vi "ConfigurationFileWriteCase.vi"() -> ()   [LabVIEW 2016]
uses:
  <vilib>/Utility/config.llb/NI_LVConfig.lvlib
  <vilib>/Utility/config.llb/Write Key (String).vi
  <vilib>/Utility/config.llb/Write Key (Boolean).vi
  <vilib>/Utility/config.llb/Write Key (Path).vi
  <vilib>/Utility/config.llb/Write Key (Double).vi
  controls/Enum.ctl
  <vilib>/Utility/config.llb/Write Key (U32).vi
  <vilib>/Utility/config.llb/Write Key (I32).vi
panel:
  in  "default name":path=path "Configuration File3.ini"
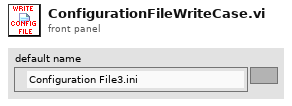
[diagram p1: front panel]
types:
  T1 = enum16{"General", "WindowPositions", "Calibration", "ZController", "Motor", "Waveforns", "ScanControl", "ScanMonitor", "Signals", "Ramp"}
  T2 = typedef "NI_LVConfig.lvlib/Config Data RefNum.ctl" = refnum<k1>
  T3 = typedef "Enum.ctl" = enum16{"Init", "Read", "Write"}
  T4 = enum16{"fractional", "engineering", "exponential"}
  T5 = enum16{"Vert. Deflection", "Horiz. Deflection", "Amplitude", "..."}
  T6 = enum32{"No Selection", "FullScale", "Standard Deviation"}
  T7 = cluster{i32, "Direction":enum16{"Forward", "Backward"}, "Processing":enum16{"None", "Offset", "Line", "Polynom"}, "Color":enum16{"Blue", "Gray", "Gold", "Green", "Red", "Asylum", "Adrian", "Nanoscope", "NanoscopeIII"}}
  T8 = enum32{"Invalid", "Standard", "Closed", "Hidden", "Minimized", "Maximized"}
  T9 = typedef "LVPositionTypeDef.ctl" = cluster{"Left":i32, "Top":i32}
  T10 = cluster{"calibName":string[], "calibParameters":cluster{"Sensitivity":cluster{"Sens X":dbl, "Sens Y":dbl, "Sens Z":dbl}, "Range":cluster{"Range X":dbl, "Range Y":dbl, "Range Z":dbl}, "HV gain":cluster{"HV gain X":dbl, "HV gain Y":dbl, "HV gain Z":dbl}}[], "calibIndex":i32}
  T11 = cluster{"Sensitivity":cluster{"Sens X":dbl, "Sens Y":dbl, "Sens Z":dbl}, "Range":cluster{"Range X":dbl, "Range Y":dbl, "Range Z":dbl}, "HV gain":cluster{"HV gain X":dbl, "HV gain Y":dbl, "HV gain Z":dbl}}[]
  T12 = cluster{"Sensitivity":cluster{"Sens X":dbl, "Sens Y":dbl, "Sens Z":dbl}, "Range":cluster{"Range X":dbl, "Range Y":dbl, "Range Z":dbl}, "HV gain":cluster{"HV gain X":dbl, "HV gain Y":dbl, "HV gain Z":dbl}}
  T13 = cluster{"Sens X":dbl, "Sens Y":dbl, "Sens Z":dbl}
  T14 = cluster{"Range X":dbl, "Range Y":dbl, "Range Z":dbl}
  T15 = cluster{"HV gain X":dbl, "HV gain Y":dbl, "HV gain Z":dbl}
  T16 = cluster{"ActiveController":dbl, "ControllerNames":string[], "ControllerParameters":cluster{"Controller Config":cluster{"Slope":bool, "Controller type":enum16{"Bipolar", "Absolute"}, "Controller name":string, "Control Signal name":string, "Signal":enum16{"Vert. Deflection", "Horiz. Deflection", "Amplitude", "..."}, "Unit":string}, "PID":cluster{"Setpoint":dbl, "P Gain":dbl, "I Gain":dbl}}[]}
  T17 = cluster{"Controller Config":cluster{"Slope":bool, "Controller type":enum16{"Bipolar", "Absolute"}, "Controller name":string, "Control Signal name":string, "Signal":enum16{"Vert. Deflection", "Horiz. Deflection", "Amplitude", "..."}, "Unit":string}, "PID":cluster{"Setpoint":dbl, "P Gain":dbl, "I Gain":dbl}}[]
  T18 = cluster{"Slope":bool, "Controller type":enum16{"Bipolar", "Absolute"}, "Controller name":string, "Control Signal name":string, "Signal":enum16{"Vert. Deflection", "Horiz. Deflection", "Amplitude", "..."}, "Unit":string}
  T19 = cluster{"Setpoint":dbl, "P Gain":dbl, "I Gain":dbl}
  T20 = typedef "ScanWaveform.ctl" = enum16{"Sine Wave", "Triangle Wave", "Rounded Wave"}
  T21 = cluster{"slowWavePts":u16, "fastWavePts":u16, "slowWaveType":T20, "fastWaveType":T20, "slowRoundPts":u16, "fastRoundPts":u16, "singleDirectionScan":bool}
  T22 = cluster{"Width":dbl, "Height":dbl, "X Offset":dbl, "Y Offset":dbl, "Angle":dbl, "Pixels/Line":u16, "Lines":u16, "Time/Line":dbl, "Scan Rate":dbl}
  T23 = enum16{"Blue", "Gray", "Gold", "Green", "Red", "Asylum", "Adrian", "Nanoscope", "NanoscopeIII"}
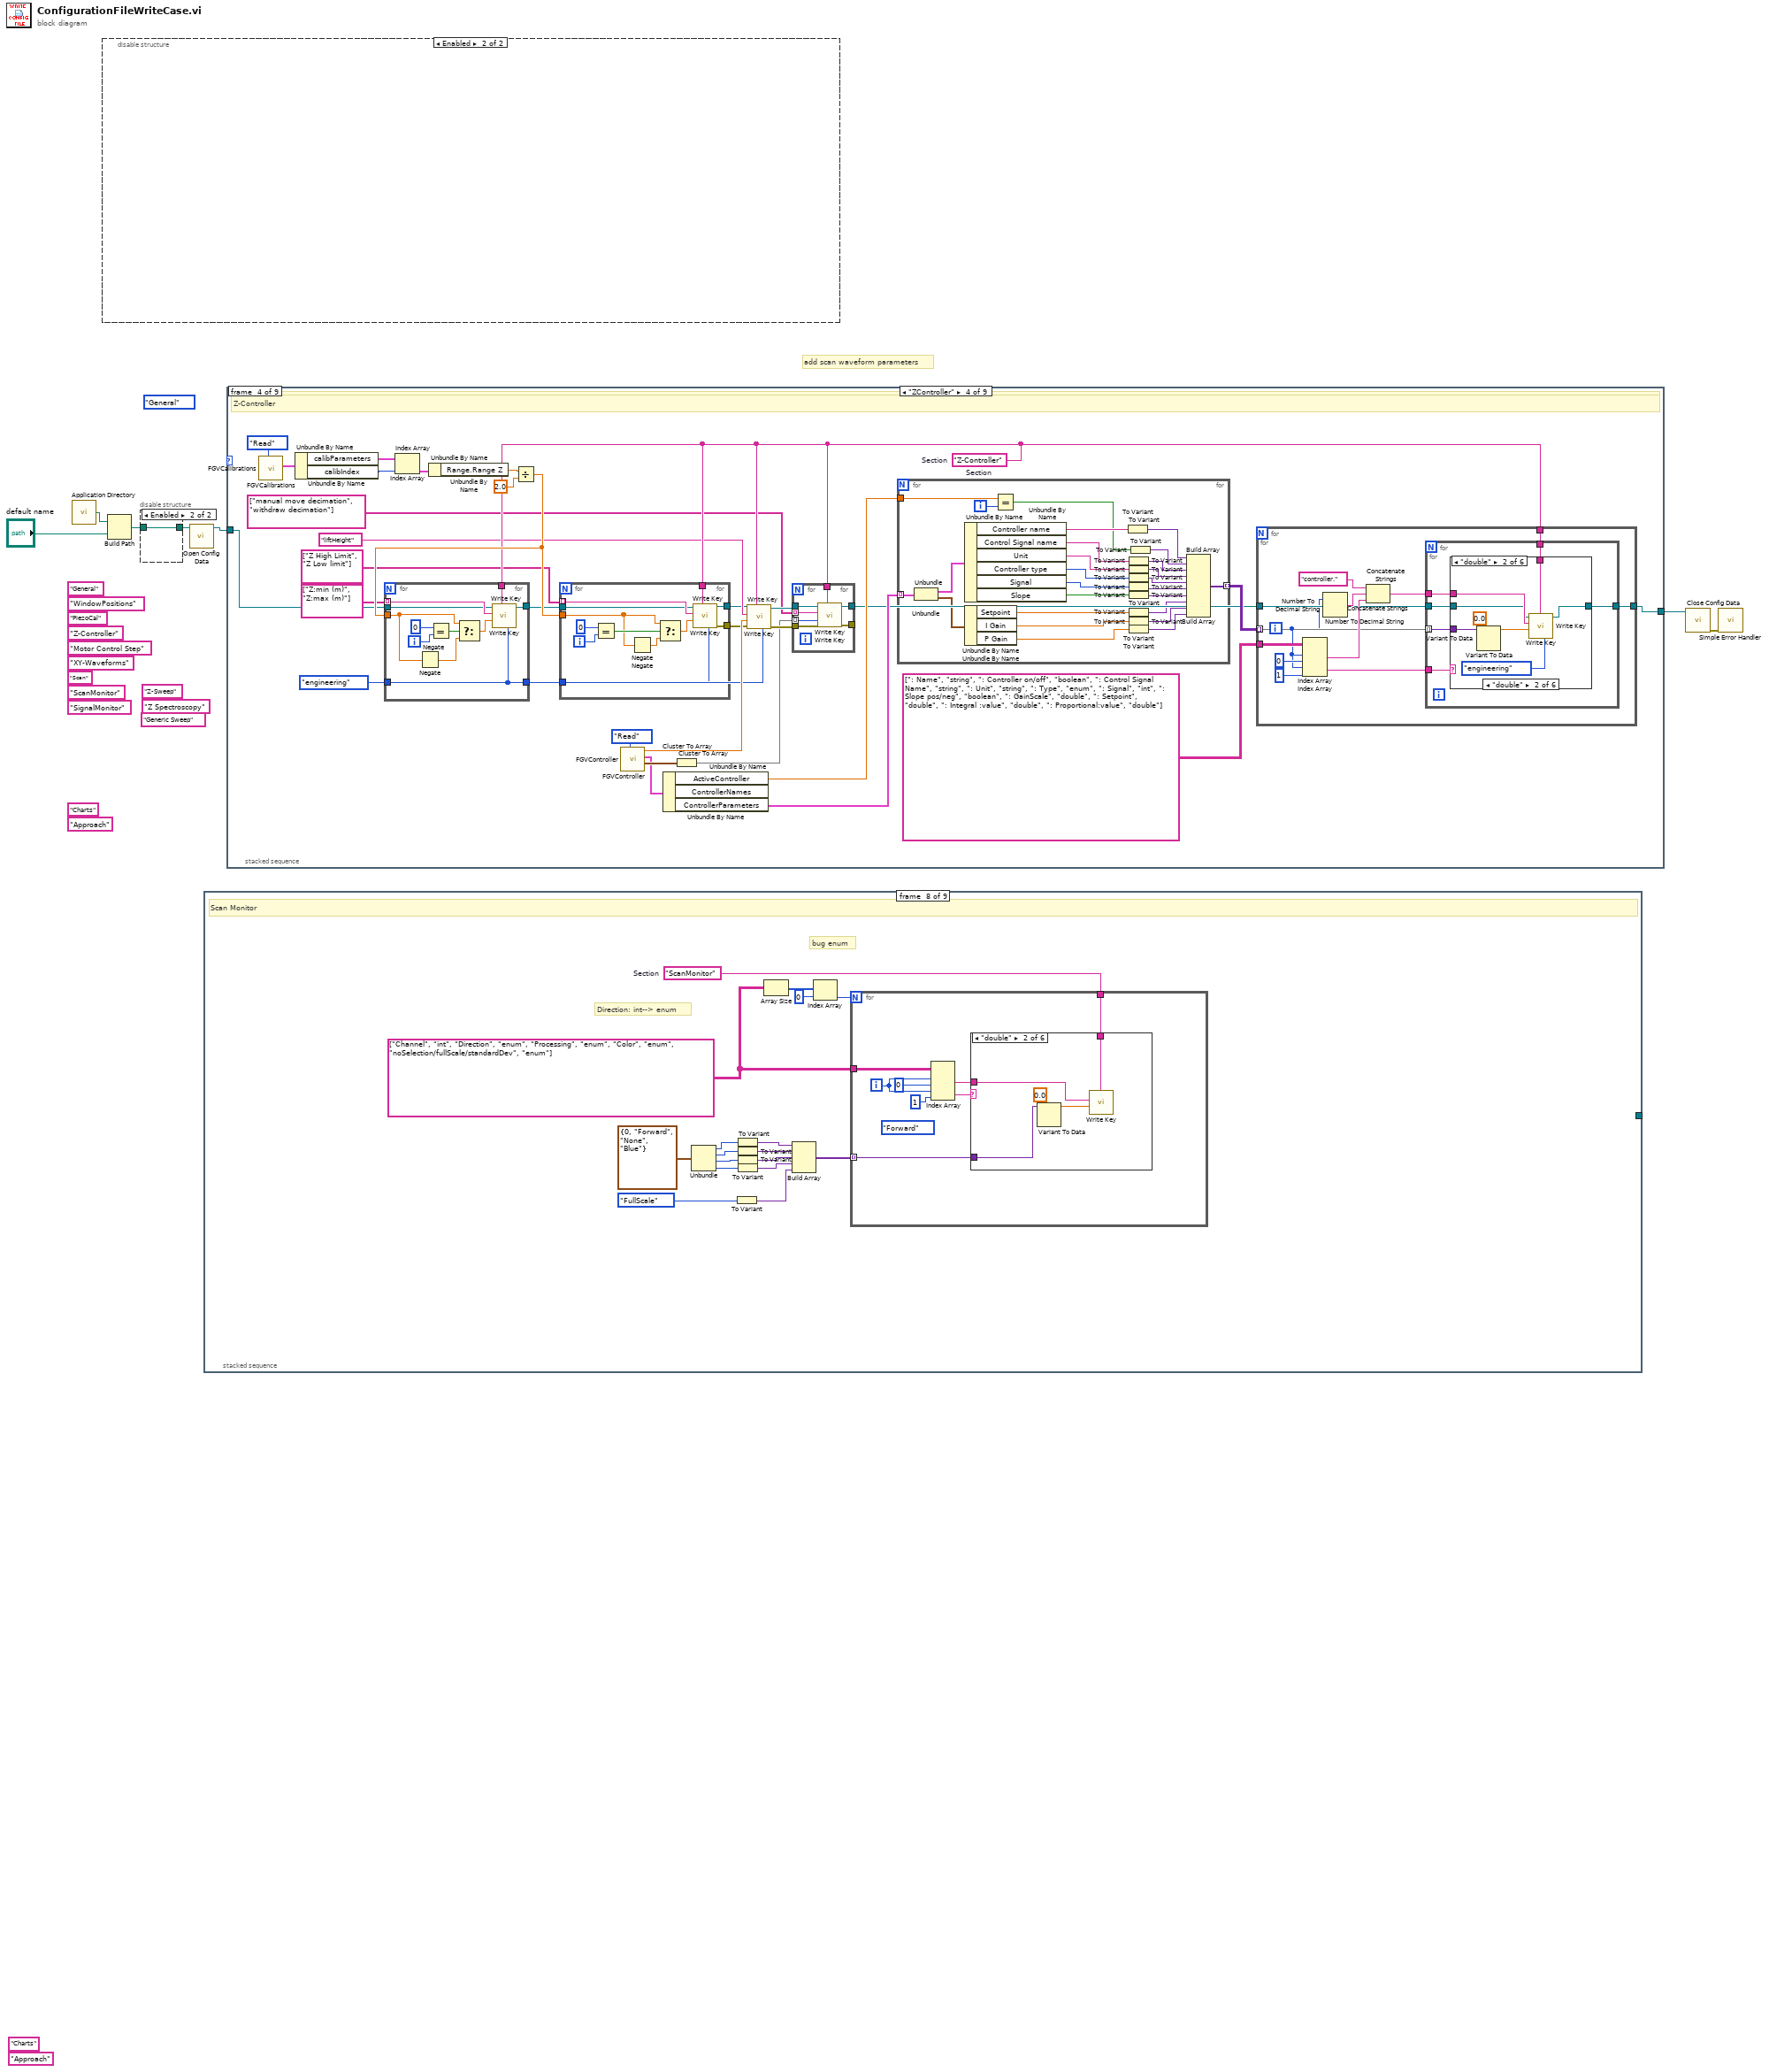
[diagram p0: block diagram]
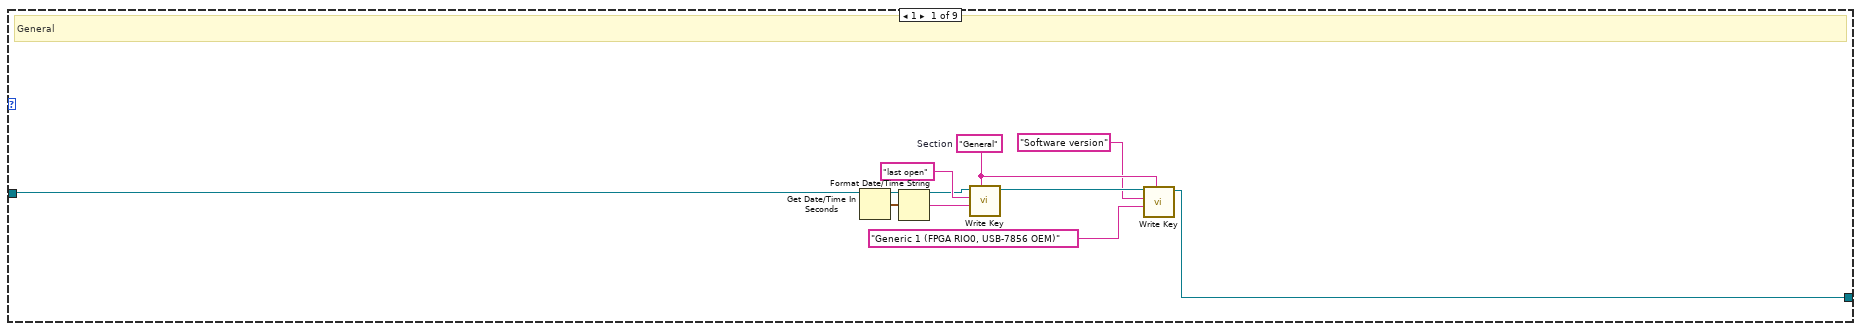
[diagram p2: hidden frame]
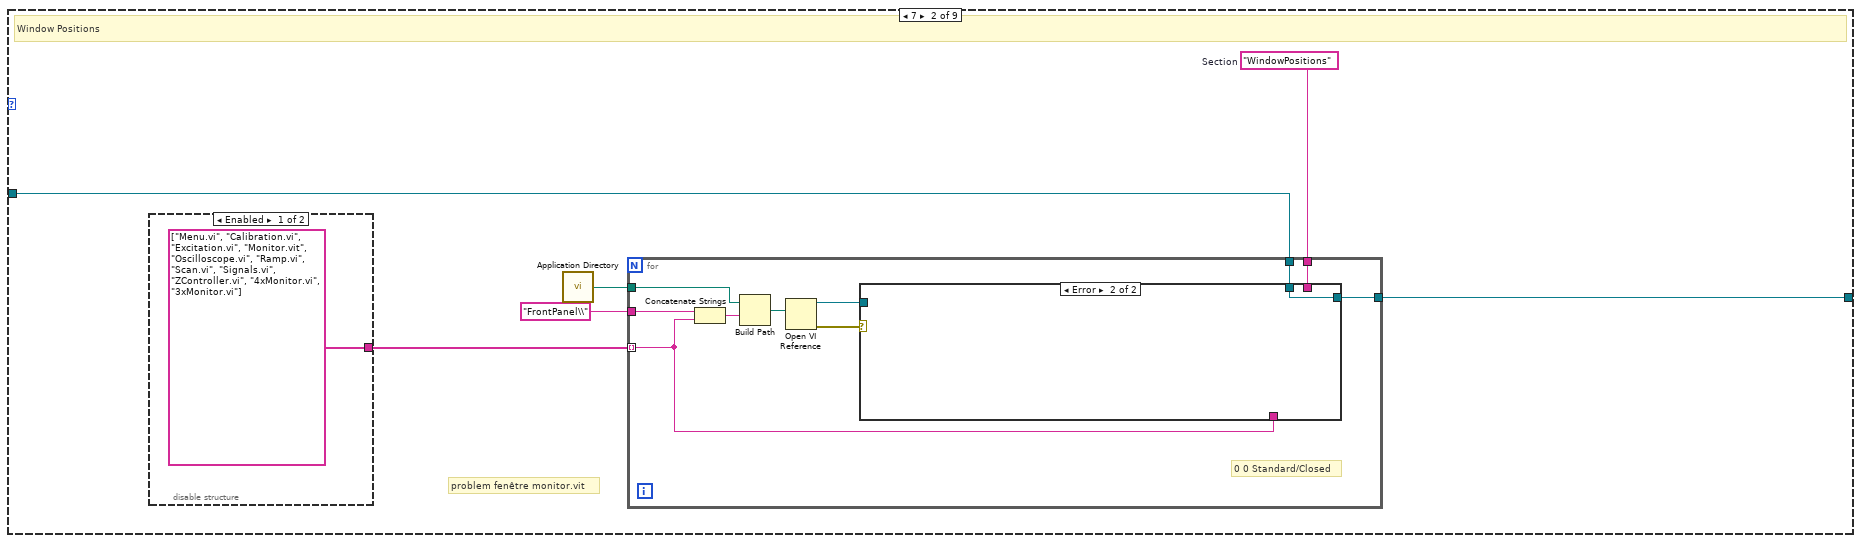
[diagram p3: hidden frame]
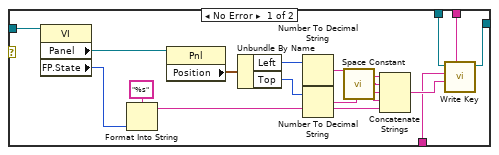
[diagram p5: hidden frame]
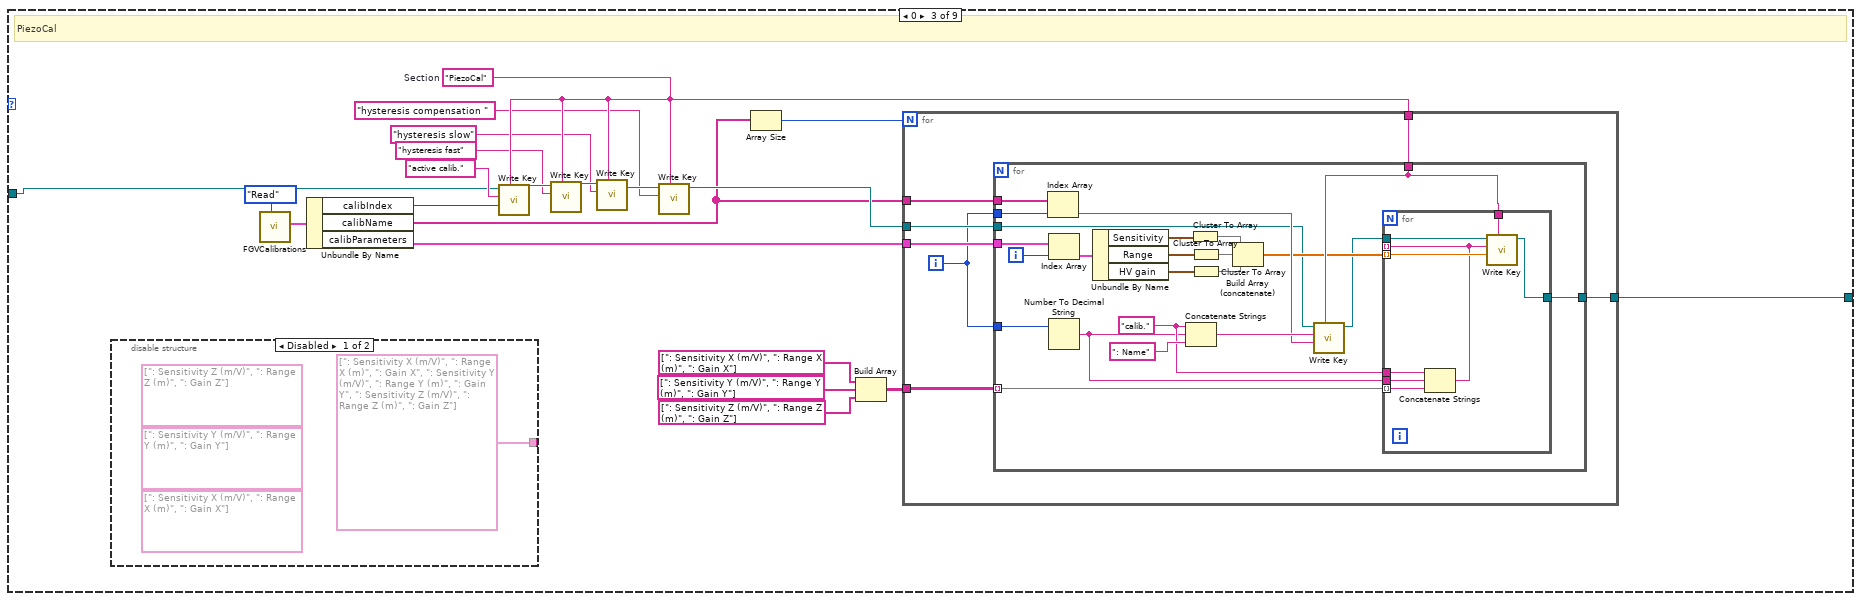
[diagram p6: hidden frame]
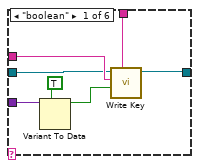
[diagram p8: hidden frame]
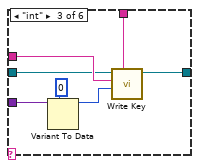
[diagram p9: hidden frame]
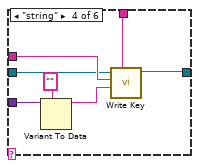
[diagram p10: hidden frame]
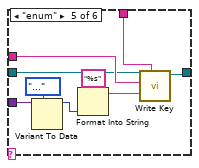
[diagram p11: hidden frame]
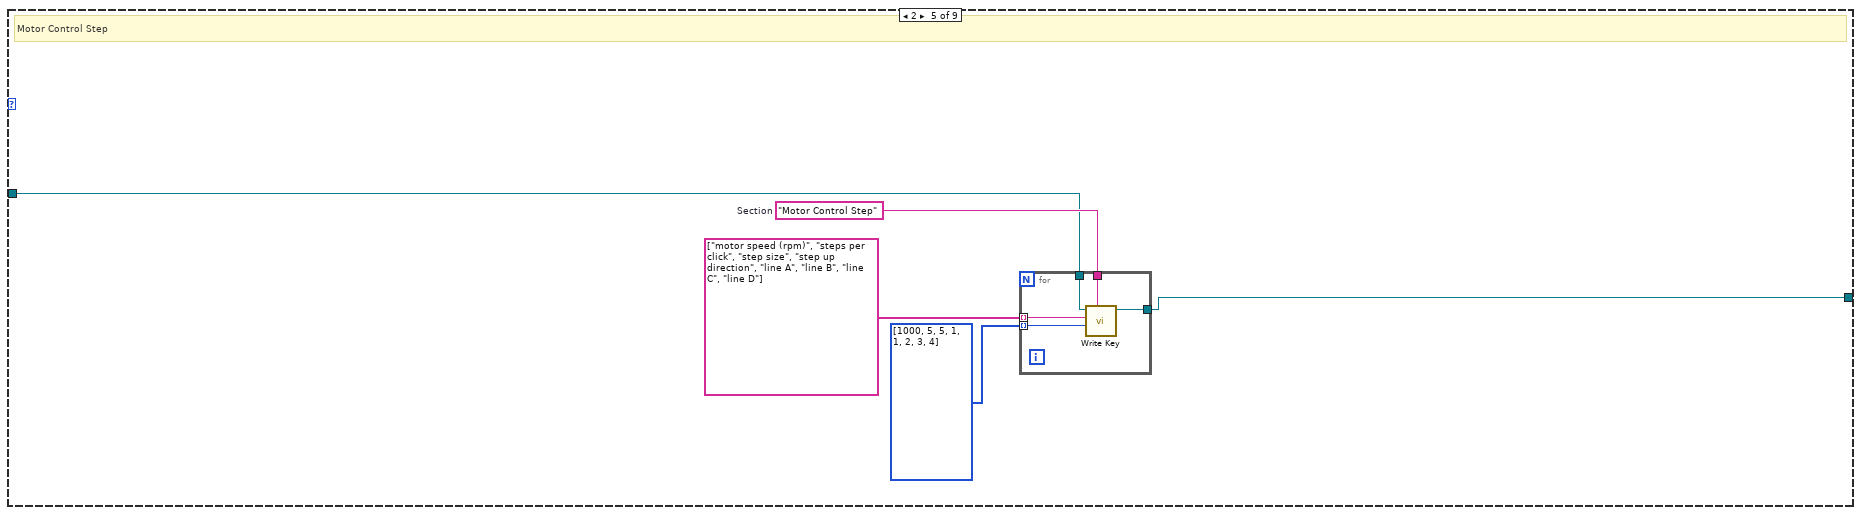
[diagram p13: hidden frame]
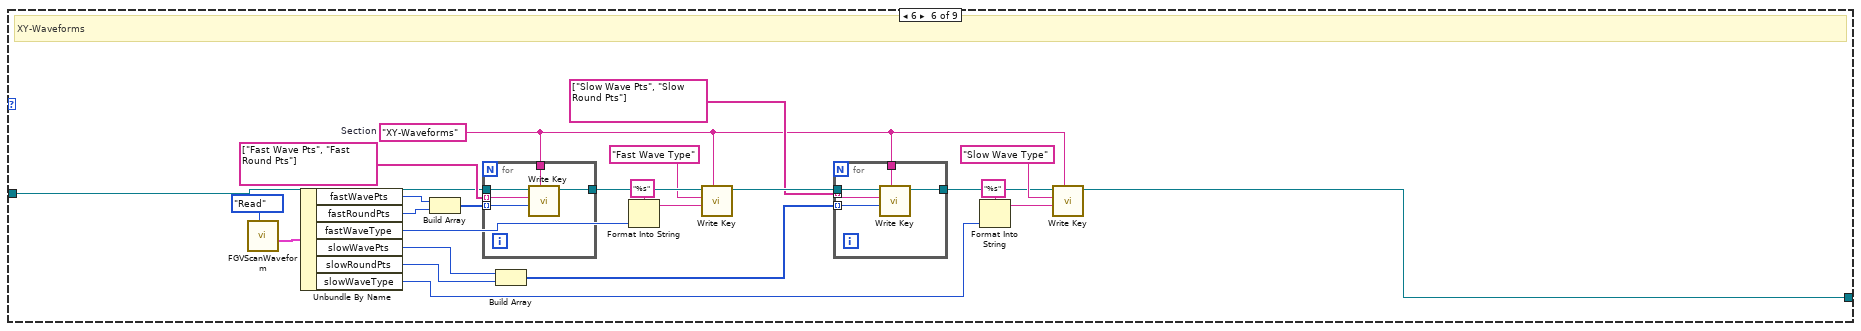
[diagram p14: hidden frame]
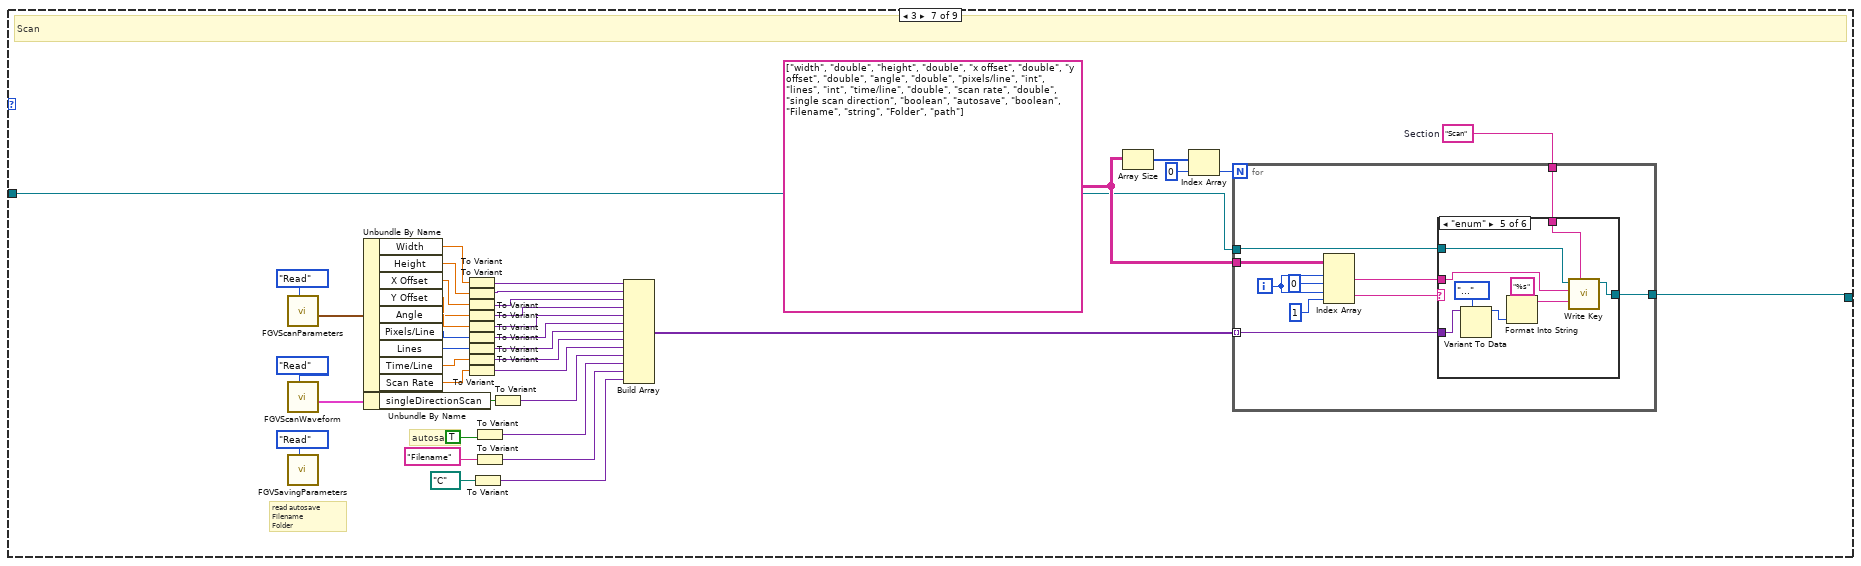
[diagram p15: hidden frame]
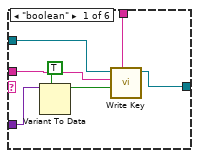
[diagram p16: hidden frame]
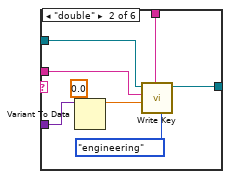
[diagram p17: hidden frame]
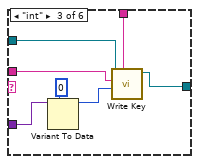
[diagram p18: hidden frame]
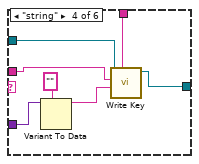
[diagram p19: hidden frame]
diagram:
  (unwired) T1."General"
  (unwired) "XY-Waveforms"
  (unwired) "Approach"
  (unwired) "Charts"
  (unwired) "Generic Sweep"
  (unwired) "ScanMonitor"
  (unwired) "Z Spectroscopy"
  (unwired) "Z-Sweep"
  (unwired) "SignalMonitor"
  (unwired) "Approach"
  (unwired) "Charts"
  (unwired) "Scan"
  (unwired) "Motor Control Step"
  (unwired) "Z-Controller"
  (unwired) "PiezoCal"
  (unwired) "WindowPositions"
  (unwired) "General"
  # "add scan waveform parameters"
  n1 = call <vilib>:"Application Directory.vi"() -> ("Application Directory"=w7:path)
  n2 = disable-structure shown="Enabled" {
    frame Disabled {
      w19 = "Second Data String"  # String 2 Value
      w20 = "First\nData\nString"  # String 1 Value
      w15 = path "C:/a/b/c.txt"  # Path Value
      w14 = 2.0  # Numeric Value
      w13 = TRUE  # Boolean Value
      w8 = FALSE  # write raw string? (F)
      w21 = "String2"  # Key 5
      w22 = "String1"  # Key 4
      w23 = "Path"  # Key 3
      w24 = "Double"  # Key 2
      w25 = "Boolean"  # Key 1
      w16 = "Section 2"
      w17 = "Section 1"
      # "string"
      # "path"
      # "boolean"
      # "double"
      n3 = call-poly <vilib>:"Write Key.vi"() -> ()  [unwired: 8 in, 4 out]
      n4 = call-poly <vilib>:"Write Key.vi"() -> ()  [unwired: 6 in, 6 out]
      n5 = call-poly <vilib>:"Write Key.vi"() -> ()  [unwired: 5 in, 7 out]
      n6 = call <vilib>:"Dflt Data Dir.vi"() -> ("App:Default Data Directory"=w11:path)
      n7 = Build Path(base path=w11, name or relative path=path "Configuration File.ini" ("default name")) -> (appended path=w9:path)
      n8 = call-poly <vilib>:"Write Key.vi"() -> ()  [unwired: 5 in, 7 out]
      n9 = Delete(path (use dialog)=w9) -> (deleted path=w10:path)  [unwired: 4 in, 2 out]
      n10 = call <vilib>:"Open Config Data.vi"("configuration file path"=w10) -> ("error out"=w30:errorcluster, "refnum"=w35:T2)  [unwired: 2 in, 7 out]
      n11 = call-poly <vilib>:"Write Key.vi"("section"=w17, "error in (no error)"=w30, "value"=w13, "key"=w25, "refnum"=w35) -> ("error out"=w29:errorcluster, "refnum out"=w34:T2)  [unwired: 5 out]
      n12 = call-poly <vilib>:"Write Key.vi"("section"=w17, "error in (no error)"=w29, "value"=w14, "key"=w24, "refnum"=w34) -> ("error out"=w28:errorcluster, "refnum out"=w33:T2)  [unwired: 3 in, 2 out]
      n13 = call-poly <vilib>:"Write Key.vi"("section"=w17, "error in (no error)"=w28, "value"=w15, "key"=w23, "refnum"=w33) -> ()  [unwired: 7 out]
      n14 = call-poly <vilib>:"Write Key.vi"("write raw string? (F)"=w8, "section"=w16, "value"=w20, "key"=w22) -> ("error out"=w27:errorcluster, "refnum out"=w32:T2)  [unwired: 2 in, 4 out]
      n15 = call-poly <vilib>:"Write Key.vi"("write raw string? (F)"=w8, "section"=w16, "error in (no error)"=w27, "value"=w19, "key"=w21, "refnum"=w32) -> ("error out"=w26:errorcluster, "refnum out"=w31:T2)  [unwired: 4 out]
      n16 = call <vilib>:"Close Config Data.vi"("error in (no error)"=w26, "refnum"=w31) -> ("error out"=w18:errorcluster)  [unwired: 1 in, 8 out]
      n17 = call <vilib>:"Simple Error Handler.vi"("error in (no error)"=w18) -> ()  [unwired: 1 in, 8 out]
    }
    frame Enabled {
    }
  }
  n18 = Build Path(base path=w7, name or relative path="default name") -> (appended path=w4:path)
  n19 = disable-structure shown="Enabled" {
    disable-tunnel: w4 -> [w37 w38]
    disable-tunnel: [w36 w38] -> w3
    frame Disabled {
      n20 = Delete(path (use dialog)=w37) -> (deleted path=w36:path)  [unwired: 4 in, 2 out]
    }
    frame Enabled {
    }
  }
  n21 = call <vilib>:"Open Config Data.vi"("configuration file path"=w3) -> ("refnum"=w1:T2)  [unwired: 2 in, 8 out]
  n22 = stacked-sequence {
    tunnel: [_ _ _ _ _ _ _ _ w434] -> _
    frame #0 {
      w45 = "General"  # Section
      # "General"
      n23 = Get Date/Time In Seconds() -> (seconds since 1Jan1904=w43:timestamp)
      n24 = Format Date/Time String(seconds (now)=w43) -> (date/time string=w44:string)  [unwired: 2 in]
      n25 = call-poly <vilib>:"Write Key.vi"("section"=w45, "value"=w44, "key"="last open") -> ("refnum out"=w42:T2)  [unwired: 3 in, 5 out]
      n26 = call-poly <vilib>:"Write Key.vi"("section"=w45, "value"="Generic 1 (FPGA RIO0, USB-7856 OEM)", "key"="Software version", "refnum"=w42) -> ()  [unwired: 2 in, 6 out]
    }
    frame #1 {
      w49 = "WindowPositions"  # Section
      # "problem fenêtre monitor.vit"
      # "Window Positions"
      n27 = disable-structure shown="Enabled" {
        disable-tunnel: [string[] ["Menu.vi", "Calibration.vi", "Excitation.vi", "Monitor.vit", "Oscilloscope.vi", "Ramp.vi", "Scan.vi", "Signals.vi", "ZController.vi", "4xMonitor.vi", "3xMonitor.vi"] _] -> w46
        frame Enabled {
        }
        frame Disabled {
        }
      }
      n28 = call <vilib>:"Application Directory.vi"() -> ("Application Directory"=w48:path)
      n29 = for {
        tunnel: "FrontPanel\\" ("string") -> [w58]
        tunnel: w48 -> [w55]
        tunnel: w46 -> [w54] mode=indexing
        tunnel: w49 -> [w53]
        # "0 0 Standard/Closed"
        n30 = Concatenate Strings(w58, w54) -> (w57:string)
        n31 = Build Path(base path=w55, name or relative path=w57) -> (appended path=w56:path)
        n32 = Open VI Reference(vi path=w56) -> (vi reference=w52:refnum<vi>, error out=w51:errorcluster)  [unwired: 5 in]
        n33 = case shown="No Error" w51 {
          tunnel: w54 -> [w65 _]
          tunnel: w53 -> [w64 _]
          tunnel: w52 -> [w63 _]
          frame No Error {
            n34 = property class="VI"(reference=w63) -> ("Panel"=w72:refnum<vi>, "FP.State"=w62:T8)  [unwired: 1 in, 2 out]
            n35 = Format Into String(format string="%s", w62) -> (resulting string=w59:string)  [unwired: 2 in, 1 out]
            n36 = property class="Pnl"(reference=w72) -> ("Position"=w71:T9)  [unwired: 1 in, 2 out]
            n37 = Unbundle By Name(w71) -> ("Left"=w70:i32, "Top"=w69:i32)
            n38 = Number To Decimal String(number=w70) -> (decimal integer string=w68:string)  [unwired: 1 in]
            n39 = Number To Decimal String(number=w69) -> (decimal integer string=w67:string)  [unwired: 1 in]
            n40 = call <vilib>:"Space Constant.vi"() -> ("String"=w60:string)
            n41 = Concatenate Strings(w68, w60, w67, w60, w59) -> (w66:string)
            n42 = call-poly <vilib>:"Write Key.vi"("section"=w64, "value"=w66, "key"=w65) -> ()  [unwired: 3 in, 6 out]
          }
          frame Error {
          }
        }
      }
    }
    frame #2 {
      w89 = "PiezoCal"  # Section
      # "PiezoCal"
      n43 = disable-structure shown="Disabled" {
        disable-tunnel: [string[] [": Sensitivity X (m/V)", ": Range X (m)", ": Gain X", ": Sensitivity Y (m/V)", ": Range Y (m)", ": Gain Y", ": Sensitivity Z (m/V)", ": Range Z (m)", ": Gain Z"] ("Array") _] -> _
        frame Disabled {
          (unwired) string[] [": Sensitivity X (m/V)", ": Range X (m)", ": Gain X"] ("Array")
          (unwired) string[] [": Sensitivity Z (m/V)", ": Range Z (m)", ": Gain Z"] ("Array")
          (unwired) string[] [": Sensitivity Y (m/V)", ": Range Y (m)", ": Gain Y"] ("Array")
        }
        frame Enabled {
        }
      }
      n44 = call "FGVCalibrations.vi"("Enum"=Enum."Read") -> ("calibOut"=w81:T10)  [unwired: 9 in, 1 out]
      n45 = Unbundle By Name(w81) -> ("calibIndex"=w91:i32, "calibName"=w77:string[], "calibParameters"=w90:T11)
      n46 = call-poly <vilib>:"Write Key.vi"("section"=w89, "value"=w91, "key"="active calib.") -> ("refnum out"=w88:T2)  [unwired: 5 in, 3 out]
      n47 = call-poly <vilib>:"Write Key.vi"("section"=w89, "key"="hysteresis fast", "refnum"=w88) -> ("refnum out"=w87:T2)  [unwired: 2 in, 6 out]
      n48 = call-poly <vilib>:"Write Key.vi"("section"=w89, "key"="hysteresis slow", "refnum"=w87) -> ("refnum out"=w86:T2)  [unwired: 2 in, 6 out]
      n49 = call-poly <vilib>:"Write Key.vi"("section"=w89, "key"="hysteresis compensation ", "refnum"=w86) -> ("refnum out"=w79:T2)  [unwired: 2 in, 6 out]
      n50 = Array Size(array=w77) -> (size(s)=w78:i32)
      n51 = Build Array(string[] [": Sensitivity X (m/V)", ": Range X (m)", ": Gain X"] ("Array"), string[] [": Sensitivity Y (m/V)", ": Range Y (m)", ": Gain Y"] ("Array"), string[] [": Sensitivity Z (m/V)", ": Range Z (m)", ": Gain Z"] ("Array")) -> (w76:string[][])
      n52 = for {
        N: w78 -> [_]
        tunnel: w90 -> [w98]
        tunnel: w76 -> [w97]
        tunnel: w89 -> [w96]
        tunnel: w77 -> [w94]
        tunnel: w79 -> [w95]
        i -> [w93]
        n53 = for {
          tunnel: w94 -> [w120]
          tunnel: w98 -> [w116]
          tunnel: w96 -> [w114]
          tunnel: w97 -> [w99] mode=indexing
          tunnel: w95 -> [w106]
          tunnel: w93 -> [w104]
          tunnel: w93 -> [w103]
          i -> [w102]
          w101 = "calib."
          n54 = Index Array(array=w120, index=w103) -> (element=w117:string)
          n55 = Index Array(array=w116, index=w102) -> (element=w115:T12)
          n56 = Number To Decimal String(number=w104) -> (decimal integer string=w100:string)  [unwired: 1 in]
          n57 = Unbundle By Name(w115) -> ("Sensitivity"=w113:T13, "Range"=w111:T14, "HV gain"=w112:T15)
          n58 = Concatenate Strings(w101, w100, ": Name") -> (w118:string)
          n59 = Cluster To Array(cluster=w113) -> (array=w110:dbl[])
          n60 = Cluster To Array(cluster=w111) -> (array=w109:dbl[])
          n61 = Cluster To Array(cluster=w112) -> (array=w108:dbl[])
          n62 = Build Array (concatenate)(w110, w109, w108) -> (w107:dbl[])
          n63 = call-poly <vilib>:"Write Key.vi"("section"=w114, "value"=w117, "key"=w118, "refnum"=w106) -> ("refnum out"=w105:T2)  [unwired: 2 in, 5 out]
          n64 = for {
            tunnel: [w121] -> _ mode=indexing
            tunnel: w114 -> [w127]
            tunnel: w107 -> [w126] mode=indexing
            tunnel: w105 -> [w125]
            tunnel: w101 -> [w124]
            tunnel: w100 -> [w123]
            tunnel: w99 -> [w122] mode=indexing
            n65 = Concatenate Strings(w124, w123, w122) -> (w121:string)
            n66 = call-poly <vilib>:"Write Key.vi"("section"=w127, "value"=w126, "key"=w121, "refnum"=w125) -> ()  [unwired: 4 in, 4 out]
          }
        }
      }
    }
    frame #3 {
      w148 = "Z-Controller"  # Section
      # "Z-Controller"
      n67 = call "FGVCalibrations.vi"("Enum"=Enum."Read") -> ("calibOut"=w151:T10)  [unwired: 9 in, 1 out]
      n68 = Unbundle By Name(w151) -> ("calibParameters"=w152:T11, "calibIndex"=w153:i32)
      n69 = Index Array(array=w152, index=w153) -> (element=w132:T12)
      n70 = Unbundle By Name(w132) -> ("Range.Range Z"=w131:dbl)
      n71 = Divide(x=w131, y=2.0) -> (x/y=w157:dbl)
      n72 = for {
        tunnel: string[] ["Z:min (m)", "Z:max (m)"] -> [w266] mode=indexing
        tunnel: w157 -> [w264]
        tunnel: w148 -> [w263]
        tunnel: [w262] -> w136
        tunnel: T4."engineering" ("format (fractional)") -> [w261]
        tunnel: [w261] -> w128
        i -> [w268]
        n73 = Negate(x=w264) -> (-x=w265:dbl)
        n74 = Equal?(x=0, y=w268) -> (x = y?=w269:bool)
        n75 = Select(t=w264, s=w269, f=w265) -> (s? t:f=w270:dbl)
        n76 = call-poly <vilib>:"Write Key.vi"("format (fractional)"=w261, "section"=w263, "value"=w270, "key"=w266) -> ("refnum out"=w262:T2)  [unwired: 4 in, 3 out]
      }
      n77 = for {
        tunnel: string[] ["Z High Limit", "Z Low limit"] -> [w256] mode=indexing
        tunnel: w157 -> [w254]
        tunnel: w148 -> [w253]
        tunnel: [w252] -> w145
        tunnel: w136 -> [w251]
        tunnel: [w250] -> w142
        tunnel: w128 -> [w249]
        i -> [w258]
        n78 = Equal?(x=0, y=w258) -> (x = y?=w259:bool)
        n79 = Negate(x=w254) -> (-x=w255:dbl)
        n80 = Select(t=w254, s=w259, f=w255) -> (s? t:f=w260:dbl)
        n81 = call-poly <vilib>:"Write Key.vi"("format (fractional)"=w249, "section"=w253, "value"=w260, "key"=w256, "refnum"=w251) -> ("error out"=w250:errorcluster, "refnum out"=w252:T2)  [unwired: 3 in, 2 out]
      }
      n82 = call "FGVController.vi"("Enum"=Enum."Read") -> ("ManualMotionDecOut"=w140:cluster{"WithdrawDec":u16, "ManualMoveDec":u16}, "calibOut"=w138:T16, "liftHeightOut"=w147:dbl)  [unwired: 6 in, 2 out]
      n83 = Unbundle By Name(w138) -> ("ActiveController"=w154:dbl, "ControllerParameters"=w155:T17)  [unwired: 1 out]
      n84 = Cluster To Array(cluster=w140) -> (array=w141:u16[])
      n85 = call-poly <vilib>:"Write Key.vi"("format (fractional)"=w128, "section"=w148, "error in (no error)"=w142, "value"=w147, "key"="liftHeight", "refnum"=w145) -> ("error out"=w143:errorcluster, "refnum out"=w144:T2)  [unwired: 2 in, 2 out]
      n86 = for {
        tunnel: w148 -> [w190]
        tunnel: w144 -> [w189]
        tunnel: w143 -> [w188]
        tunnel: string[] ["manual move decimation", "withdraw decimation"] -> [w187] mode=indexing
        tunnel: w141 -> [w186] mode=indexing
        tunnel: [w185] -> _
        tunnel: [w184] -> w130
        n87 = call-poly <vilib>:"Write Key.vi"("section"=w190, "error in (no error)"=w188, "value"=w186, "key"=w187, "refnum"=w189) -> ("error out"=w185:errorcluster, "refnum out"=w184:T2)  [unwired: 3 in, 2 out]
      }
      n88 = for {
        tunnel: w155 -> [w183] mode=indexing
        tunnel: w154 -> [w161]
        tunnel: [w158] -> w149 mode=indexing
        i -> [w162]
        n89 = Unbundle(w183) -> ("Controller Config"=w182:T18, "PID"=w181:T19)
        n90 = Unbundle By Name(w182) -> ("Controller name"=w180:string, "Control Signal name"=w179:string, "Unit"=w178:string, "Controller type"=w177:enum16{"Bipolar", "Absolute"}, "Signal"=w176:T5, "Slope"=w175:bool)
        n91 = Unbundle By Name(w181) -> ("Setpoint"=w174:dbl, "I Gain"=w173:dbl, "P Gain"=w172:dbl)
        n92 = Equal?(x=w161, y=w162) -> (x = y?=w160:bool)
        n93 = To Variant(anything=w180) -> (Variant=w171:variant)
        n94 = To Variant(anything=w179) -> (Variant=w170:variant)
        n95 = To Variant(anything=w178) -> (Variant=w169:variant)
        n96 = To Variant(anything=w177) -> (Variant=w168:variant)
        n97 = To Variant(anything=w176) -> (Variant=w167:variant)
        n98 = To Variant(anything=w175) -> (Variant=w166:variant)
        n99 = To Variant(anything=w174) -> (Variant=w165:variant)
        n100 = To Variant(anything=w173) -> (Variant=w164:variant)
        n101 = To Variant(anything=w172) -> (Variant=w163:variant)
        n102 = To Variant(anything=w160) -> (Variant=w159:variant)
        n103 = Build Array(w171, w159, w170, w169, w168, w167, w166, w165, w164, w163) -> (w158:variant[])
      }
      n104 = for {
        tunnel: string[][] [[": Name", "string"], [": Controller on/off", "boolean"], [": Control Signal Name", "string"], [": Unit", "string"], [": Type", "enum"], [": Signal", "int"], [": Slope pos/neg", "boolean"], [": GainScale", "double"], [": Setpoint", "double"], [": Integral :value", "double"], [": Proportional:value", "double"]] ("appended array") -> [w199]
        tunnel: w149 -> [w194] mode=indexing
        tunnel: w148 -> [w196]
        tunnel: w130 -> [w192]
        tunnel: [w193] -> _
        i -> [w191]
        n105 = Index Array(array=w199, index (row) #1=w191, index (col) #1=0 ("disabled index (col)"), index (row) #2=w191, index (col) #2=1 ("disabled index (col)")) -> (element #1=w201:string, element #2=w197:string)
        n106 = Number To Decimal String(number=w191) -> (decimal integer string=w202:string)  [unwired: 1 in]
        n107 = Concatenate Strings("controller.", w202, w201) -> (w195:string)
        n108 = for {
          tunnel: w197 -> [w209]
          tunnel: w196 -> [w208]
          tunnel: w195 -> [w207]
          tunnel: w194 -> [w206] mode=indexing
          tunnel: w192 -> [w204]
          tunnel: [w205] -> w193
          n109 = case shown="\"double\"" w209 {
            tunnel: w208 -> [w213 w220 w227 w238 w247 _]
            tunnel: w207 -> [w212 w221 w228 w237 w246 _]
            tunnel: w206 -> [w216 w223 w230 w234 w245 _]
            tunnel: [w210 w218 w226 w233 w239 w248] -> w205
            tunnel: w204 -> [w211 w219 w225 w232 w240 w248]
            frame "boolean" {
              n110 = Variant To Data(type=TRUE, Variant=w216) -> (data=w214:bool)  [unwired: 1 in, 1 out]
              n111 = call-poly <vilib>:"Write Key.vi"("section"=w213, "value"=w214, "key"=w212, "refnum"=w211) -> ("refnum out"=w210:T2)  [unwired: 1 in, 6 out]
            }
            frame "double" {
              n112 = Variant To Data(type=0.0 ("Signal"), Variant=w223) -> (data=w222:dbl)  [unwired: 1 in, 1 out]
              n113 = call-poly <vilib>:"Write Key.vi"("format (fractional)"=T4."engineering", "section"=w220, "value"=w222, "key"=w221, "refnum"=w219) -> ("refnum out"=w218:T2)  [unwired: 3 in, 3 out]
            }
            frame "int" {
              n114 = Variant To Data(type=u16 0 ("Signal"), Variant=w230) -> (data=w229:u16)  [unwired: 1 in, 1 out]
              n115 = call-poly <vilib>:"Write Key.vi"("section"=w227, "value"=w229, "key"=w228, "refnum"=w225) -> ("refnum out"=w226:T2)  [unwired: 1 in, 6 out]
            }
            frame "string" {
              n116 = Variant To Data(type="", Variant=w234) -> (data=w235:string)  [unwired: 1 in, 1 out]
              n117 = call-poly <vilib>:"Write Key.vi"("section"=w238, "value"=w235, "key"=w237, "refnum"=w232) -> ("refnum out"=w233:T2)  [unwired: 2 in, 5 out]
            }
            frame "enum" {
              n118 = Variant To Data(type=T5."..." ("Signal"), Variant=w245) -> (data=w243:T5)  [unwired: 1 in, 1 out]
              n119 = Format Into String(format string="%s", w243) -> (resulting string=w241:string)  [unwired: 2 in, 1 out]
              n120 = call-poly <vilib>:"Write Key.vi"("section"=w247, "value"=w241, "key"=w246, "refnum"=w240) -> ("refnum out"=w239:T2)  [unwired: 2 in, 5 out]
            }
            frame Default {
            }
          }
        }
      }
    }
    frame #4 {
      w273 = "Motor Control Step"  # Section
      # "Motor Control Step"
      n121 = for {
        tunnel: string[] ["motor speed (rpm)", "steps per click", "step size", "step up direction", "line A", "line B", "line C", "line D"] -> [w277] mode=indexing
        tunnel: i32[] [1000, 5, 5, 1, 1, 2, 3, 4] ("number") -> [w276] mode=indexing
        tunnel: w273 -> [w275]
        tunnel: [w274] -> _
        n122 = call-poly <vilib>:"Write Key.vi"("section"=w275, "value"=w276, "key"=w277) -> ("refnum out"=w274:T2)  [unwired: 2 in, 6 out]
      }
    }
    frame #5 {
      w281 = "XY-Waveforms"  # Section
      # "XY-Waveforms"
      n123 = call "FGVScanWaveform.vi"("Enum"=Enum."Read") -> ("scanWaveFormCtl Out"=w298:T21)  [unwired: 9 in, 1 out]
      n124 = Unbundle By Name(w298) -> ("fastWavePts"=w297:u16, "fastRoundPts"=w296:u16, "fastWaveType"=w294:T20, "slowWavePts"=w280:u16, "slowRoundPts"=w279:u16, "slowWaveType"=w278:T20)
      n125 = Build Array(w297, w296) -> (w295:u16[])
      n126 = for {
        tunnel: w295 -> [w308] mode=indexing
        tunnel: string[] ["Fast Wave Pts", "Fast Round Pts"] -> [w307] mode=indexing
        tunnel: w281 -> [w306]
        tunnel: [w305] -> w292
        n127 = call-poly <vilib>:"Write Key.vi"("section"=w306, "value"=w308, "key"=w307) -> ("refnum out"=w305:T2)  [unwired: 2 in, 6 out]
      }
      n128 = Build Array(w280, w279) -> (w283:u16[])
      n129 = Format Into String(format string="%s", w294) -> (resulting string=w291:string)  [unwired: 2 in, 1 out]
      n130 = call-poly <vilib>:"Write Key.vi"("section"=w281, "value"=w291, "key"="Fast Wave Type", "refnum"=w292) -> ("refnum out"=w284:T2)  [unwired: 2 in, 5 out]
      n131 = for {
        tunnel: w283 -> [w304] mode=indexing
        tunnel: string[] ["Slow Wave Pts", "Slow Round Pts"] -> [w303] mode=indexing
        tunnel: w281 -> [w302]
        tunnel: [w301] -> w286
        tunnel: w284 -> [w300]
        n132 = call-poly <vilib>:"Write Key.vi"("section"=w302, "value"=w304, "key"=w303, "refnum"=w300) -> ("refnum out"=w301:T2)  [unwired: 1 in, 6 out]
      }
      n133 = Format Into String(format string="%s", w278) -> (resulting string=w287:string)  [unwired: 2 in, 1 out]
      n134 = call-poly <vilib>:"Write Key.vi"("section"=w281, "value"=w287, "key"="Slow Wave Type", "refnum"=w286) -> ()  [unwired: 2 in, 6 out]
    }
    frame #6 {
      w312 = string[][] [["width", "double"], ["height", "double"], ["x offset", "double"], ["y offset", "double"], ["angle", "double"], ["pixels/line", "int"], ["lines", "int"], ["time/line", "double"], ["scan rate", "double"], ["single scan direction", "boolean"], ["autosave", "boolean"], ["Filename", "string"], ["Folder", "path"]] ("transposed array")
      w335 = "Scan"  # Section
      # "read autosave\nFilename\nFolder"
      # "autosave"
      # "Scan"
      n135 = call "FGVScanParameters.vi"("Enum"=Enum."Read") -> ("Scan Parameters Out"=w315:T22)  [unwired: 9 in, 1 out]
      n136 = call "FGVScanWaveform.vi"("Enum"=Enum."Read") -> ("scanWaveFormCtl Out"=w337:T21)  [unwired: 9 in, 1 out]
      n137 = call "FGVSavingParameters.vi"("Enum"=Enum."Read") -> ()  [unwired: 7 in, 4 out]
      n138 = Unbundle By Name(w315) -> ("Width"=w325:dbl, "Height"=w326:dbl, "X Offset"=w327:dbl, "Y Offset"=w328:dbl, "Angle"=w329:dbl, "Pixels/Line"=w330:u16, "Lines"=w331:u16, "Time/Line"=w332:dbl, "Scan Rate"=w333:dbl)
      n139 = Unbundle By Name(w337) -> ("singleDirectionScan"=w338:bool)
      n140 = To Variant(anything=w325) -> (Variant=w316:variant)
      n141 = To Variant(anything=w326) -> (Variant=w324:variant)
      n142 = To Variant(anything=w327) -> (Variant=w317:variant)
      n143 = To Variant(anything=w328) -> (Variant=w318:variant)
      n144 = To Variant(anything=w329) -> (Variant=w319:variant)
      n145 = To Variant(anything=w330) -> (Variant=w320:variant)
      n146 = To Variant(anything=w331) -> (Variant=w321:variant)
      n147 = To Variant(anything=w332) -> (Variant=w322:variant)
      n148 = To Variant(anything=w333) -> (Variant=w323:variant)
      n149 = To Variant(anything=path "C:/") -> (Variant=w345:variant)
      n150 = To Variant(anything=TRUE) -> (Variant=w343:variant)
      n151 = To Variant(anything="Filename") -> (Variant=w344:variant)
      n152 = To Variant(anything=w338) -> (Variant=w339:variant)
      n153 = Build Array(w316, w324, w317, w318, w319, w320, w321, w322, w323, w339, w343, w344, w345) -> (w334:variant[])
      n154 = Array Size(array=w312) -> (size(s)=w311:i32[])
      n155 = Index Array(array=w311, index=0) -> (element=w310:i32)
      n156 = for {
        N: w310 -> [_]
        tunnel: w312 -> [w351]
        tunnel: w334 -> [w353] mode=indexing
        tunnel: w335 -> [w352]
        i -> [w348]
        n157 = Index Array(array=w351, index (row) #1=w348, index (col) #1=0 ("disabled index (col)"), index (row) #2=w348, index (col) #2=1 ("disabled index (col)")) -> (element #1=w349:string, element #2=w346:string)
        n158 = case shown="\"double\"" w346 {
          tunnel: w353 -> [w356 w362 w367 w372 w377 _]
          tunnel: w352 -> [w355 w361 w366 w370 w376 _]
          tunnel: w349 -> [w354 w360 w365 w371 w375 _]
          frame "boolean" {
            n159 = Variant To Data(type=TRUE, Variant=w356) -> (data=w357:bool)  [unwired: 1 in, 1 out]
            n160 = call-poly <vilib>:"Write Key.vi"("section"=w355, "value"=w357, "key"=w354) -> ()  [unwired: 2 in, 7 out]
          }
          frame "double" {
            n161 = Variant To Data(type=0.0 ("Signal"), Variant=w362) -> (data=w363:dbl)  [unwired: 1 in, 1 out]
            n162 = call-poly <vilib>:"Write Key.vi"("format (fractional)"=T4."engineering", "section"=w361, "value"=w363, "key"=w360) -> ()  [unwired: 4 in, 4 out]
          }
          frame "int" {
            n163 = Variant To Data(type=u32 0 ("Signal"), Variant=w367) -> (data=w368:u32)  [unwired: 1 in, 1 out]
            n164 = call-poly <vilib>:"Write Key.vi"("section"=w366, "value"=w368, "key"=w365) -> ()  [unwired: 2 in, 7 out]
          }
          frame "string" {
            n165 = Variant To Data(type="", Variant=w372) -> (data=w373:string)  [unwired: 1 in, 1 out]
            n166 = call-poly <vilib>:"Write Key.vi"("section"=w370, "value"=w373, "key"=w371) -> ()  [unwired: 3 in, 6 out]
          }
          frame "enum" {
            n167 = Variant To Data(type=T5."..." ("Signal"), Variant=w377) -> (data=w380:T5)  [unwired: 1 in, 1 out]
            n168 = Format Into String(format string="%s", w380) -> (resulting string=w378:string)  [unwired: 2 in, 1 out]
            n169 = call-poly <vilib>:"Write Key.vi"("section"=w376, "value"=w378, "key"=w375) -> ()  [unwired: 3 in, 6 out]
          }
          frame Default {
          }
        }
      }
    }
    frame #7 {
      w385 = string[][] [["Channel", "int"], ["Direction", "enum"], ["Processing", "enum"], ["Color", "enum"], ["noSelection/fullScale/standardDev", "enum"]] ("transposed array")
      w386 = "ScanMonitor"  # Section
      # "bug enum"
      # "Direction: int--> enum"
      # "Scan Monitor"
      n170 = Unbundle(T7 {0, "Direction"=enum."Forward", "Processing"=enum."None", "Color"=enum."Blue"} ("Controls")) -> (w392:i32, "Direction"=w393:enum16{"Forward", "Backward"}, "Processing"=w394:enum16{"None", "Offset", "Line", "Polynom"}, "Color"=w395:T23)
      n171 = To Variant(anything=T6."FullScale" ("ZScale")) -> (Variant=w397:variant)
      n172 = To Variant(anything=w392) -> (Variant=w387:variant)
      n173 = To Variant(anything=w393) -> (Variant=w390:variant)
      n174 = To Variant(anything=w394) -> (Variant=w389:variant)
      n175 = To Variant(anything=w395) -> (Variant=w388:variant)
      n176 = Array Size(array=w385) -> (size(s)=w383:i32[])
      n177 = Build Array(w387, w390, w389, w388, w397) -> (w396:variant[])
      n178 = Index Array(array=w383, index=0) -> (element=w384:i32)
      n179 = for {
        N: w384 -> [_]
        tunnel: w385 -> [w405]
        tunnel: w386 -> [w406]
        tunnel: w396 -> [w399] mode=indexing
        i -> [w402]
        (unwired) enum16{"Forward", "Backward"}."Forward" ("Direction")
        n180 = Index Array(array=w405, index (row) #1=w402, index (col) #1=0 ("disabled index (col)"), index (row) #2=w402, index (col) #2=1 ("disabled index (col)")) -> (element #1=w403:string, element #2=w400:string)
        n181 = case shown="\"double\"" w400 {
          tunnel: w406 -> [w408 w412 w419 w423 w428 _]
          tunnel: w403 -> [w407 w413 w418 w422 w429 _]
          tunnel: w399 -> [w409 w414 w417 w424 w430 _]
          frame "boolean" {
            n182 = Variant To Data(type=TRUE, Variant=w409) -> (data=w410:bool)  [unwired: 1 in, 1 out]
            n183 = call-poly <vilib>:"Write Key.vi"("section"=w408, "value"=w410, "key"=w407) -> ()  [unwired: 2 in, 7 out]
          }
          frame "double" {
            n184 = Variant To Data(type=0.0 ("Signal"), Variant=w414) -> (data=w415:dbl)  [unwired: 1 in, 1 out]
            n185 = call-poly <vilib>:"Write Key.vi"("section"=w412, "value"=w415, "key"=w413) -> ()  [unwired: 5 in, 4 out]
          }
          frame "int" {
            n186 = Variant To Data(type=u32 0 ("Signal"), Variant=w417) -> (data=w420:u32)  [unwired: 1 in, 1 out]
            n187 = call-poly <vilib>:"Write Key.vi"("section"=w419, "value"=w420, "key"=w418) -> ()  [unwired: 2 in, 7 out]
          }
          frame "string" {
            n188 = Variant To Data(type="", Variant=w424) -> (data=w425:string)  [unwired: 1 in, 1 out]
            n189 = call-poly <vilib>:"Write Key.vi"("section"=w423, "value"=w425, "key"=w422) -> ()  [unwired: 3 in, 6 out]
          }
          frame "enum" {
            n190 = Variant To Data(type=enum16{""}."", Variant=w430) -> (data=w433:enum16{""})  [unwired: 1 in, 1 out]
            n191 = Format Into String(format string="%s", w433) -> (resulting string=w431:string)  [unwired: 2 in, 1 out]
            n192 = call-poly <vilib>:"Write Key.vi"("section"=w428, "value"=w431, "key"=w429) -> ()  [unwired: 3 in, 6 out]
          }
          frame Default {
          }
        }
      }
    }
    frame #8 {
      w442 = i32[] [0, 0, 0, 0, 0, 0, 0, 0]  # Offset
      w441 = i32[] [-1, 1, 1, 1, 1, 1, 1, 1]  # Cal
      w437 = string[] ["m", "V", "V", "V", "V", "V", "V", ""]  # Unit
      w435 = string[] ["Height", "Vert. Deflection", "Horiz. Deflection", "Channel 4", "Channel 5", "Channel 6", "AuxIn", "Obelix"]  # Name
      w443 = "SignalMonitor"  # Section
      # "replace by fgv Signals"
      # "Signal Monitor"
      n193 = for {
        tunnel: w435 -> [w462] mode=indexing
        tunnel: "channel " -> [w461]
        tunnel: w437 -> [w452] mode=indexing
        tunnel: "unit " -> [w459]
        tunnel: "cal " -> [w458]
        tunnel: "offset " -> [w457]
        tunnel: w441 -> [w451] mode=indexing
        tunnel: w442 -> [w450] mode=indexing
        tunnel: w443 -> [w449]
        tunnel: [w445] -> w434
        i -> [w444]
        n194 = Number To Decimal String(number=w444) -> (decimal integer string=w456:string)  [unwired: 1 in]
        n195 = Concatenate Strings(w461, w456) -> (w460:string)
        n196 = Concatenate Strings(w459, w456) -> (w455:string)
        n197 = Concatenate Strings(w458, w456) -> (w454:string)
        n198 = Concatenate Strings(w457, w456) -> (w453:string)
        n199 = call-poly <vilib>:"Write Key.vi"("section"=w449, "value"=w462, "key"=w460) -> ("refnum out"=w448:T2)  [unwired: 3 in, 5 out]
        n200 = call-poly <vilib>:"Write Key.vi"("section"=w449, "value"=w452, "key"=w455, "refnum"=w448) -> ("refnum out"=w447:T2)  [unwired: 2 in, 5 out]
        n201 = call-poly <vilib>:"Write Key.vi"("section"=w449, "value"=w451, "key"=w454, "refnum"=w447) -> ("refnum out"=w446:T2)  [unwired: 1 in, 6 out]
        n202 = call-poly <vilib>:"Write Key.vi"("section"=w449, "value"=w450, "key"=w453, "refnum"=w446) -> ("refnum out"=w445:T2)  [unwired: 1 in, 6 out]
      }
    }
  }
  n203 = case shown="\"ZController\"" {
    tunnel: [w464 w473 w507 w567 w713 w723 w757 w845 w912] -> _
    selector: _ -> [_ _ _ _ _ _ _ _ _]
    tunnel: w1 -> [w463 w472 w506 w566 w712 w722 w756 w844 w911]
    frame 1 {
      w471 = "General"  # Section
      # "General"
      n204 = Get Date/Time In Seconds() -> (seconds since 1Jan1904=w469:timestamp)
      n205 = Format Date/Time String(seconds (now)=w469) -> (date/time string=w470:string)  [unwired: 2 in]
      n206 = call-poly <vilib>:"Write Key.vi"("section"=w471, "value"=w470, "key"="last open", "refnum"=w463) -> ("refnum out"=w468:T2)  [unwired: 2 in, 5 out]
      n207 = call-poly <vilib>:"Write Key.vi"("section"=w471, "value"="Generic 1 (FPGA RIO0, USB-7856 OEM)", "key"="Software version", "refnum"=w468) -> ("refnum out"=w464:T2)  [unwired: 2 in, 5 out]
    }
    frame 7 {
      w477 = "WindowPositions"  # Section
      # "problem fenêtre monitor.vit"
      # "Window Positions"
      n208 = disable-structure shown="Enabled" {
        disable-tunnel: [string[] ["Menu.vi", "Calibration.vi", "Excitation.vi", "Monitor.vit", "Oscilloscope.vi", "Ramp.vi", "Scan.vi", "Signals.vi", "ZController.vi", "4xMonitor.vi", "3xMonitor.vi"] _] -> w474
        frame Enabled {
        }
        frame Disabled {
        }
      }
      n209 = call <vilib>:"Application Directory.vi"() -> ("Application Directory"=w476:path)
      n210 = for {
        tunnel: "FrontPanel\\" ("string") -> [w488]
        tunnel: w476 -> [w485]
        tunnel: w474 -> [w484] mode=indexing
        tunnel: w477 -> [w483]
        tunnel: [w480] -> w473
        tunnel: w472 -> [w479]
        # "0 0 Standard/Closed"
        n211 = Concatenate Strings(w488, w484) -> (w487:string)
        n212 = Build Path(base path=w485, name or relative path=w487) -> (appended path=w486:path)
        n213 = Open VI Reference(vi path=w486) -> (vi reference=w482:refnum<vi>, error out=w481:errorcluster)  [unwired: 5 in]
        n214 = case shown="Error" w481 {
          tunnel: w484 -> [w497 _]
          tunnel: w483 -> [w496 _]
          tunnel: w482 -> [w495 _]
          tunnel: [w490 w505] -> w480
          tunnel: w479 -> [w489 w505]
          frame No Error {
            n215 = property class="VI"(reference=w495) -> ("Panel"=w504:refnum<vi>, "FP.State"=w494:T8)  [unwired: 1 in, 2 out]
            n216 = Format Into String(format string="%s", w494) -> (resulting string=w491:string)  [unwired: 2 in, 1 out]
            n217 = property class="Pnl"(reference=w504) -> ("Position"=w503:T9)  [unwired: 1 in, 2 out]
            n218 = Unbundle By Name(w503) -> ("Left"=w502:i32, "Top"=w501:i32)
            n219 = Number To Decimal String(number=w502) -> (decimal integer string=w500:string)  [unwired: 1 in]
            n220 = Number To Decimal String(number=w501) -> (decimal integer string=w499:string)  [unwired: 1 in]
            n221 = call <vilib>:"Space Constant.vi"() -> ("String"=w492:string)
            n222 = Concatenate Strings(w500, w492, w499, w492, w491) -> (w498:string)
            n223 = call-poly <vilib>:"Write Key.vi"("section"=w496, "value"=w498, "key"=w497, "refnum"=w489) -> ("refnum out"=w490:T2)  [unwired: 2 in, 5 out]
          }
          frame Error {
          }
        }
      }
    }
    frame 0 {
      w524 = "PiezoCal"  # Section
      # "PiezoCal"
      n224 = disable-structure shown="Disabled" {
        disable-tunnel: [string[] [": Sensitivity X (m/V)", ": Range X (m)", ": Gain X", ": Sensitivity Y (m/V)", ": Range Y (m)", ": Gain Y", ": Sensitivity Z (m/V)", ": Range Z (m)", ": Gain Z"] ("Array") _] -> _
        frame Disabled {
          (unwired) string[] [": Sensitivity X (m/V)", ": Range X (m)", ": Gain X"] ("Array")
          (unwired) string[] [": Sensitivity Z (m/V)", ": Range Z (m)", ": Gain Z"] ("Array")
          (unwired) string[] [": Sensitivity Y (m/V)", ": Range Y (m)", ": Gain Y"] ("Array")
        }
        frame Enabled {
        }
      }
      n225 = call "FGVCalibrations.vi"("Enum"=Enum."Read") -> ("calibOut"=w516:T10)  [unwired: 9 in, 1 out]
      n226 = Unbundle By Name(w516) -> ("calibIndex"=w526:i32, "calibName"=w512:string[], "calibParameters"=w525:T11)
      n227 = call-poly <vilib>:"Write Key.vi"("section"=w524, "value"=w526, "key"="active calib.", "refnum"=w506) -> ("refnum out"=w523:T2)  [unwired: 4 in, 3 out]
      n228 = call-poly <vilib>:"Write Key.vi"("section"=w524, "key"="hysteresis fast", "refnum"=w523) -> ("refnum out"=w522:T2)  [unwired: 2 in, 6 out]
      n229 = call-poly <vilib>:"Write Key.vi"("section"=w524, "key"="hysteresis slow", "refnum"=w522) -> ("refnum out"=w521:T2)  [unwired: 2 in, 6 out]
      n230 = call-poly <vilib>:"Write Key.vi"("section"=w524, "key"="hysteresis compensation ", "refnum"=w521) -> ("refnum out"=w514:T2)  [unwired: 2 in, 6 out]
      n231 = Array Size(array=w512) -> (size(s)=w513:i32)
      n232 = Build Array(string[] [": Sensitivity X (m/V)", ": Range X (m)", ": Gain X"] ("Array"), string[] [": Sensitivity Y (m/V)", ": Range Y (m)", ": Gain Y"] ("Array"), string[] [": Sensitivity Z (m/V)", ": Range Z (m)", ": Gain Z"] ("Array")) -> (w511:string[][])
      n233 = for {
        N: w513 -> [_]
        tunnel: w525 -> [w534]
        tunnel: w511 -> [w533]
        tunnel: w524 -> [w532]
        tunnel: w512 -> [w530]
        tunnel: w514 -> [w531]
        tunnel: [w528] -> w507
        i -> [w529]
        n234 = for {
          tunnel: w530 -> [w557]
          tunnel: w534 -> [w553]
          tunnel: w532 -> [w551]
          tunnel: w533 -> [w536] mode=indexing
          tunnel: w531 -> [w543]
          tunnel: w529 -> [w541]
          tunnel: w529 -> [w540]
          tunnel: [w535] -> w528
          i -> [w539]
          w538 = "calib."
          n235 = Index Array(array=w557, index=w540) -> (element=w554:string)
          n236 = Index Array(array=w553, index=w539) -> (element=w552:T12)
          n237 = Number To Decimal String(number=w541) -> (decimal integer string=w537:string)  [unwired: 1 in]
          n238 = Unbundle By Name(w552) -> ("Sensitivity"=w550:T13, "Range"=w548:T14, "HV gain"=w549:T15)
          n239 = Concatenate Strings(w538, w537, ": Name") -> (w555:string)
          n240 = Cluster To Array(cluster=w550) -> (array=w547:dbl[])
          n241 = Cluster To Array(cluster=w548) -> (array=w546:dbl[])
          n242 = Cluster To Array(cluster=w549) -> (array=w545:dbl[])
          n243 = Build Array (concatenate)(w547, w546, w545) -> (w544:dbl[])
          n244 = call-poly <vilib>:"Write Key.vi"("section"=w551, "value"=w554, "key"=w555, "refnum"=w543) -> ("refnum out"=w542:T2)  [unwired: 2 in, 5 out]
          n245 = for {
            tunnel: [w559] -> _ mode=indexing
            tunnel: w551 -> [w565]
            tunnel: w544 -> [w564] mode=indexing
            tunnel: w542 -> [w563]
            tunnel: w538 -> [w562]
            tunnel: w537 -> [w561]
            tunnel: w536 -> [w560] mode=indexing
            tunnel: [w558] -> w535
            n246 = Concatenate Strings(w562, w561, w560) -> (w559:string)
            n247 = call-poly <vilib>:"Write Key.vi"("section"=w565, "value"=w564, "key"=w559, "refnum"=w563) -> ("refnum out"=w558:T2)  [unwired: 4 in, 3 out]
          }
        }
      }
    }
    frame 8 {
      w588 = "Z-Controller"  # Section
      # "Z-Controller"
      n248 = call "FGVCalibrations.vi"("Enum"=Enum."Read") -> ("calibOut"=w591:T10)  [unwired: 9 in, 1 out]
      n249 = Unbundle By Name(w591) -> ("calibParameters"=w592:T11, "calibIndex"=w593:i32)
      n250 = Index Array(array=w592, index=w593) -> (element=w572:T12)
      n251 = Unbundle By Name(w572) -> ("Range.Range Z"=w571:dbl)
      n252 = Divide(x=w571, y=2.0) -> (x/y=w597:dbl)
      n253 = for {
        tunnel: string[] ["Z:min (m)", "Z:max (m)"] -> [w707] mode=indexing
        tunnel: w597 -> [w705]
        tunnel: w588 -> [w704]
        tunnel: [w703] -> w576
        tunnel: T4."engineering" ("format (fractional)") -> [w702]
        tunnel: [w702] -> w568
        tunnel: w566 -> [w701]
        i -> [w709]
        n254 = Negate(x=w705) -> (-x=w706:dbl)
        n255 = Equal?(x=0, y=w709) -> (x = y?=w710:bool)
        n256 = Select(t=w705, s=w710, f=w706) -> (s? t:f=w711:dbl)
        n257 = call-poly <vilib>:"Write Key.vi"("format (fractional)"=w702, "section"=w704, "value"=w711, "key"=w707, "refnum"=w701) -> ("refnum out"=w703:T2)  [unwired: 3 in, 3 out]
      }
      n258 = for {
        tunnel: string[] ["Z High Limit", "Z Low limit"] -> [w696] mode=indexing
        tunnel: w597 -> [w694]
        tunnel: w588 -> [w693]
        tunnel: [w692] -> w585
        tunnel: w576 -> [w691]
        tunnel: [w690] -> w582
        tunnel: w568 -> [w689]
        i -> [w698]
        n259 = Equal?(x=0, y=w698) -> (x = y?=w699:bool)
        n260 = Negate(x=w694) -> (-x=w695:dbl)
        n261 = Select(t=w694, s=w699, f=w695) -> (s? t:f=w700:dbl)
        n262 = call-poly <vilib>:"Write Key.vi"("format (fractional)"=w689, "section"=w693, "value"=w700, "key"=w696, "refnum"=w691) -> ("error out"=w690:errorcluster, "refnum out"=w692:T2)  [unwired: 3 in, 2 out]
      }
      n263 = call "FGVController.vi"("Enum"=Enum."Read") -> ("ManualMotionDecOut"=w580:cluster{"WithdrawDec":u16, "ManualMoveDec":u16}, "calibOut"=w578:T16, "liftHeightOut"=w587:dbl)  [unwired: 6 in, 2 out]
      n264 = Unbundle By Name(w578) -> ("ActiveController"=w594:dbl, "ControllerParameters"=w595:T17)  [unwired: 1 out]
      n265 = Cluster To Array(cluster=w580) -> (array=w581:u16[])
      n266 = call-poly <vilib>:"Write Key.vi"("format (fractional)"=w568, "section"=w588, "error in (no error)"=w582, "value"=w587, "key"="liftHeight", "refnum"=w585) -> ("error out"=w583:errorcluster, "refnum out"=w584:T2)  [unwired: 2 in, 2 out]
      n267 = for {
        tunnel: w588 -> [w630]
        tunnel: w584 -> [w629]
        tunnel: w583 -> [w628]
        tunnel: string[] ["manual move decimation", "withdraw decimation"] -> [w627] mode=indexing
        tunnel: w581 -> [w626] mode=indexing
        tunnel: [w625] -> _
        tunnel: [w624] -> w570
        n268 = call-poly <vilib>:"Write Key.vi"("section"=w630, "error in (no error)"=w628, "value"=w626, "key"=w627, "refnum"=w629) -> ("error out"=w625:errorcluster, "refnum out"=w624:T2)  [unwired: 3 in, 2 out]
      }
      n269 = for {
        tunnel: w595 -> [w623] mode=indexing
        tunnel: w594 -> [w601]
        tunnel: [w598] -> w589 mode=indexing
        i -> [w602]
        n270 = Unbundle(w623) -> ("Controller Config"=w622:T18, "PID"=w621:T19)
        n271 = Unbundle By Name(w622) -> ("Controller name"=w620:string, "Control Signal name"=w619:string, "Unit"=w618:string, "Controller type"=w617:enum16{"Bipolar", "Absolute"}, "Signal"=w616:T5, "Slope"=w615:bool)
        n272 = Unbundle By Name(w621) -> ("Setpoint"=w614:dbl, "I Gain"=w613:dbl, "P Gain"=w612:dbl)
        n273 = Equal?(x=w601, y=w602) -> (x = y?=w600:bool)
        n274 = To Variant(anything=w620) -> (Variant=w611:variant)
        n275 = To Variant(anything=w619) -> (Variant=w610:variant)
        n276 = To Variant(anything=w618) -> (Variant=w609:variant)
        n277 = To Variant(anything=w617) -> (Variant=w608:variant)
        n278 = To Variant(anything=w616) -> (Variant=w607:variant)
        n279 = To Variant(anything=w615) -> (Variant=w606:variant)
        n280 = To Variant(anything=w614) -> (Variant=w605:variant)
        n281 = To Variant(anything=w613) -> (Variant=w604:variant)
        n282 = To Variant(anything=w612) -> (Variant=w603:variant)
        n283 = To Variant(anything=w600) -> (Variant=w599:variant)
        n284 = Build Array(w611, w599, w610, w609, w608, w607, w606, w605, w604, w603) -> (w598:variant[])
      }
      n285 = for {
        tunnel: string[][] [[": Name", "string"], [": Controller on/off", "boolean"], [": Control Signal Name", "string"], [": Unit", "string"], [": Type", "enum"], [": Signal", "int"], [": Slope pos/neg", "boolean"], [": GainScale", "double"], [": Setpoint", "double"], [": Integral :value", "double"], [": Proportional:value", "double"]] ("appended array") -> [w639]
        tunnel: w589 -> [w634] mode=indexing
        tunnel: w588 -> [w636]
        tunnel: w570 -> [w632]
        tunnel: [w633] -> w567
        i -> [w631]
        n286 = Index Array(array=w639, index (row) #1=w631, index (col) #1=0 ("disabled index (col)"), index (row) #2=w631, index (col) #2=1 ("disabled index (col)")) -> (element #1=w641:string, element #2=w637:string)
        n287 = Number To Decimal String(number=w631) -> (decimal integer string=w642:string)  [unwired: 1 in]
        n288 = Concatenate Strings("controller.", w642, w641) -> (w635:string)
        n289 = for {
          tunnel: w637 -> [w649]
          tunnel: w636 -> [w648]
          tunnel: w635 -> [w647]
          tunnel: w634 -> [w646] mode=indexing
          tunnel: w632 -> [w644]
          tunnel: [w645] -> w633
          n290 = case shown="\"double\"" w649 {
            tunnel: w648 -> [w653 w660 w667 w678 w687 _]
            tunnel: w647 -> [w652 w661 w668 w677 w686 _]
            tunnel: w646 -> [w656 w663 w670 w674 w685 _]
            tunnel: [w650 w658 w666 w673 w679 w688] -> w645
            tunnel: w644 -> [w651 w659 w665 w672 w680 w688]
            frame "boolean" {
              n291 = Variant To Data(type=TRUE, Variant=w656) -> (data=w654:bool)  [unwired: 1 in, 1 out]
              n292 = call-poly <vilib>:"Write Key.vi"("section"=w653, "value"=w654, "key"=w652, "refnum"=w651) -> ("refnum out"=w650:T2)  [unwired: 1 in, 6 out]
            }
            frame "double" {
              n293 = Variant To Data(type=0.0 ("Signal"), Variant=w663) -> (data=w662:dbl)  [unwired: 1 in, 1 out]
              n294 = call-poly <vilib>:"Write Key.vi"("format (fractional)"=T4."engineering", "section"=w660, "value"=w662, "key"=w661, "refnum"=w659) -> ("refnum out"=w658:T2)  [unwired: 3 in, 3 out]
            }
            frame "int" {
              n295 = Variant To Data(type=u16 0 ("Signal"), Variant=w670) -> (data=w669:u16)  [unwired: 1 in, 1 out]
              n296 = call-poly <vilib>:"Write Key.vi"("section"=w667, "value"=w669, "key"=w668, "refnum"=w665) -> ("refnum out"=w666:T2)  [unwired: 1 in, 6 out]
            }
            frame "string" {
              n297 = Variant To Data(type="", Variant=w674) -> (data=w675:string)  [unwired: 1 in, 1 out]
              n298 = call-poly <vilib>:"Write Key.vi"("section"=w678, "value"=w675, "key"=w677, "refnum"=w672) -> ("refnum out"=w673:T2)  [unwired: 2 in, 5 out]
            }
            frame "enum" {
              n299 = Variant To Data(type=T5."..." ("Signal"), Variant=w685) -> (data=w683:T5)  [unwired: 1 in, 1 out]
              n300 = Format Into String(format string="%s", w683) -> (resulting string=w681:string)  [unwired: 2 in, 1 out]
              n301 = call-poly <vilib>:"Write Key.vi"("section"=w687, "value"=w681, "key"=w686, "refnum"=w680) -> ("refnum out"=w679:T2)  [unwired: 2 in, 5 out]
            }
            frame Default {
            }
          }
        }
      }
    }
    frame 2 {
      w716 = "Motor Control Step"  # Section
      # "Motor Control Step"
      n302 = for {
        tunnel: string[] ["motor speed (rpm)", "steps per click", "step size", "step up direction", "line A", "line B", "line C", "line D"] -> [w721] mode=indexing
        tunnel: i32[] [1000, 5, 5, 1, 1, 2, 3, 4] ("number") -> [w720] mode=indexing
        tunnel: w716 -> [w719]
        tunnel: [w718] -> w713
        tunnel: w712 -> [w717]
        n303 = call-poly <vilib>:"Write Key.vi"("section"=w719, "value"=w720, "key"=w721, "refnum"=w717) -> ("refnum out"=w718:T2)  [unwired: 1 in, 6 out]
      }
    }
    frame 6 {
      w727 = "XY-Waveforms"  # Section
      # "XY-Waveforms"
      n304 = call "FGVScanWaveform.vi"("Enum"=Enum."Read") -> ("scanWaveFormCtl Out"=w744:T21)  [unwired: 9 in, 1 out]
      n305 = Unbundle By Name(w744) -> ("fastWavePts"=w743:u16, "fastRoundPts"=w742:u16, "fastWaveType"=w740:T20, "slowWavePts"=w726:u16, "slowRoundPts"=w725:u16, "slowWaveType"=w724:T20)
      n306 = Build Array(w743, w742) -> (w741:u16[])
      n307 = for {
        tunnel: w741 -> [w755] mode=indexing
        tunnel: string[] ["Fast Wave Pts", "Fast Round Pts"] -> [w754] mode=indexing
        tunnel: w727 -> [w753]
        tunnel: [w752] -> w738
        tunnel: w722 -> [w751]
        n308 = call-poly <vilib>:"Write Key.vi"("section"=w753, "value"=w755, "key"=w754, "refnum"=w751) -> ("refnum out"=w752:T2)  [unwired: 1 in, 6 out]
      }
      n309 = Build Array(w726, w725) -> (w729:u16[])
      n310 = Format Into String(format string="%s", w740) -> (resulting string=w737:string)  [unwired: 2 in, 1 out]
      n311 = call-poly <vilib>:"Write Key.vi"("section"=w727, "value"=w737, "key"="Fast Wave Type", "refnum"=w738) -> ("refnum out"=w730:T2)  [unwired: 2 in, 5 out]
      n312 = for {
        tunnel: w729 -> [w750] mode=indexing
        tunnel: string[] ["Slow Wave Pts", "Slow Round Pts"] -> [w749] mode=indexing
        tunnel: w727 -> [w748]
        tunnel: [w747] -> w732
        tunnel: w730 -> [w746]
        n313 = call-poly <vilib>:"Write Key.vi"("section"=w748, "value"=w750, "key"=w749, "refnum"=w746) -> ("refnum out"=w747:T2)  [unwired: 1 in, 6 out]
      }
      n314 = Format Into String(format string="%s", w724) -> (resulting string=w733:string)  [unwired: 2 in, 1 out]
      n315 = call-poly <vilib>:"Write Key.vi"("section"=w727, "value"=w733, "key"="Slow Wave Type", "refnum"=w732) -> ("refnum out"=w723:T2)  [unwired: 2 in, 5 out]
    }
    frame 3 {
      w761 = string[][] [["width", "double"], ["height", "double"], ["x offset", "double"], ["y offset", "double"], ["angle", "double"], ["pixels/line", "int"], ["lines", "int"], ["time/line", "double"], ["scan rate", "double"], ["single scan direction", "boolean"], ["autosave", "boolean"], ["Filename", "string"], ["Folder", "path"]] ("transposed array")
      w784 = "Scan"  # Section
      # "read autosave\nFilename\nFolder"
      # "autosave"
      # "Scan"
      n316 = call "FGVScanParameters.vi"("Enum"=Enum."Read") -> ("Scan Parameters Out"=w764:T22)  [unwired: 9 in, 1 out]
      n317 = call "FGVScanWaveform.vi"("Enum"=Enum."Read") -> ("scanWaveFormCtl Out"=w786:T21)  [unwired: 9 in, 1 out]
      n318 = call "FGVSavingParameters.vi"("Enum"=Enum."Read") -> ()  [unwired: 7 in, 4 out]
      n319 = Unbundle By Name(w764) -> ("Width"=w774:dbl, "Height"=w775:dbl, "X Offset"=w776:dbl, "Y Offset"=w777:dbl, "Angle"=w778:dbl, "Pixels/Line"=w779:u16, "Lines"=w780:u16, "Time/Line"=w781:dbl, "Scan Rate"=w782:dbl)
      n320 = Unbundle By Name(w786) -> ("singleDirectionScan"=w787:bool)
      n321 = To Variant(anything=w774) -> (Variant=w765:variant)
      n322 = To Variant(anything=w775) -> (Variant=w773:variant)
      n323 = To Variant(anything=w776) -> (Variant=w766:variant)
      n324 = To Variant(anything=w777) -> (Variant=w767:variant)
      n325 = To Variant(anything=w778) -> (Variant=w768:variant)
      n326 = To Variant(anything=w779) -> (Variant=w769:variant)
      n327 = To Variant(anything=w780) -> (Variant=w770:variant)
      n328 = To Variant(anything=w781) -> (Variant=w771:variant)
      n329 = To Variant(anything=w782) -> (Variant=w772:variant)
      n330 = To Variant(anything=path "C:/") -> (Variant=w794:variant)
      n331 = To Variant(anything=TRUE) -> (Variant=w792:variant)
      n332 = To Variant(anything="Filename") -> (Variant=w793:variant)
      n333 = To Variant(anything=w787) -> (Variant=w788:variant)
      n334 = Build Array(w765, w773, w766, w767, w768, w769, w770, w771, w772, w788, w792, w793, w794) -> (w783:variant[])
      n335 = Array Size(array=w761) -> (size(s)=w760:i32[])
      n336 = Index Array(array=w760, index=0) -> (element=w759:i32)
      n337 = for {
        N: w759 -> [_]
        tunnel: w761 -> [w802]
        tunnel: w783 -> [w804] mode=indexing
        tunnel: w784 -> [w803]
        tunnel: [w796] -> w757
        tunnel: w756 -> [w795]
        i -> [w799]
        n338 = Index Array(array=w802, index (row) #1=w799, index (col) #1=0 ("disabled index (col)"), index (row) #2=w799, index (col) #2=1 ("disabled index (col)")) -> (element #1=w800:string, element #2=w797:string)
        n339 = case shown="\"enum\"" w797 {
          tunnel: w804 -> [w809 w817 w824 w831 w838 _]
          tunnel: w803 -> [w808 w816 w823 w829 w837 _]
          tunnel: w800 -> [w807 w815 w822 w830 w836 _]
          tunnel: [w806 w813 w821 w828 w835 w843] -> w796
          tunnel: w795 -> [w805 w812 w820 w827 w834 w843]
          frame "boolean" {
            n340 = Variant To Data(type=TRUE, Variant=w809) -> (data=w810:bool)  [unwired: 1 in, 1 out]
            n341 = call-poly <vilib>:"Write Key.vi"("section"=w808, "value"=w810, "key"=w807, "refnum"=w805) -> ("refnum out"=w806:T2)  [unwired: 1 in, 6 out]
          }
          frame "double" {
            n342 = Variant To Data(type=0.0 ("Signal"), Variant=w817) -> (data=w818:dbl)  [unwired: 1 in, 1 out]
            n343 = call-poly <vilib>:"Write Key.vi"("format (fractional)"=T4."engineering", "section"=w816, "value"=w818, "key"=w815, "refnum"=w812) -> ("refnum out"=w813:T2)  [unwired: 3 in, 3 out]
          }
          frame "int" {
            n344 = Variant To Data(type=u32 0 ("Signal"), Variant=w824) -> (data=w825:u32)  [unwired: 1 in, 1 out]
            n345 = call-poly <vilib>:"Write Key.vi"("section"=w823, "value"=w825, "key"=w822, "refnum"=w820) -> ("refnum out"=w821:T2)  [unwired: 1 in, 6 out]
          }
          frame "string" {
            n346 = Variant To Data(type="", Variant=w831) -> (data=w832:string)  [unwired: 1 in, 1 out]
            n347 = call-poly <vilib>:"Write Key.vi"("section"=w829, "value"=w832, "key"=w830, "refnum"=w827) -> ("refnum out"=w828:T2)  [unwired: 2 in, 5 out]
          }
          frame "enum" {
            n348 = Variant To Data(type=T5."..." ("Signal"), Variant=w838) -> (data=w841:T5)  [unwired: 1 in, 1 out]
            n349 = Format Into String(format string="%s", w841) -> (resulting string=w839:string)  [unwired: 2 in, 1 out]
            n350 = call-poly <vilib>:"Write Key.vi"("section"=w837, "value"=w839, "key"=w836, "refnum"=w834) -> ("refnum out"=w835:T2)  [unwired: 2 in, 5 out]
          }
          frame Default {
          }
        }
      }
    }
    frame 4 {
      w849 = string[][] [["Channel", "int"], ["Direction", "enum"], ["Processing", "enum"], ["Color", "enum"], ["noSelection/fullScale/standardDev", "enum"]] ("transposed array")
      w850 = "ScanMonitor"  # Section
      # "bug enum"
      # "Direction: int--> enum"
      # "Scan Monitor"
      n351 = Unbundle(T7 {0, "Direction"=enum."Forward", "Processing"=enum."None", "Color"=enum."Blue"} ("Controls")) -> (w856:i32, "Direction"=w857:enum16{"Forward", "Backward"}, "Processing"=w858:enum16{"None", "Offset", "Line", "Polynom"}, "Color"=w859:T23)
      n352 = To Variant(anything=T6."FullScale" ("ZScale")) -> (Variant=w861:variant)
      n353 = To Variant(anything=w856) -> (Variant=w851:variant)
      n354 = To Variant(anything=w857) -> (Variant=w854:variant)
      n355 = To Variant(anything=w858) -> (Variant=w853:variant)
      n356 = To Variant(anything=w859) -> (Variant=w852:variant)
      n357 = Array Size(array=w849) -> (size(s)=w847:i32[])
      n358 = Build Array(w851, w854, w853, w852, w861) -> (w860:variant[])
      n359 = Index Array(array=w847, index=0) -> (element=w848:i32)
      n360 = for {
        N: w848 -> [_]
        tunnel: w849 -> [w871]
        tunnel: w850 -> [w872]
        tunnel: w860 -> [w865] mode=indexing
        tunnel: [w864] -> w845
        tunnel: w844 -> [w863]
        i -> [w868]
        (unwired) enum16{"Forward", "Backward"}."Forward" ("Direction")
        n361 = Index Array(array=w871, index (row) #1=w868, index (col) #1=0 ("disabled index (col)"), index (row) #2=w868, index (col) #2=1 ("disabled index (col)")) -> (element #1=w869:string, element #2=w866:string)
        n362 = case shown="Default" w866 {
          tunnel: w872 -> [w876 w882 w891 w897 w904 _]
          tunnel: w869 -> [w875 w883 w890 w896 w905 _]
          tunnel: w865 -> [w877 w884 w889 w898 w906 _]
          tunnel: [w874 w881 w888 w895 w902 w910] -> w864
          tunnel: w863 -> [w873 w880 w887 w894 w901 w910]
          frame "boolean" {
            n363 = Variant To Data(type=TRUE, Variant=w877) -> (data=w878:bool)  [unwired: 1 in, 1 out]
            n364 = call-poly <vilib>:"Write Key.vi"("section"=w876, "value"=w878, "key"=w875, "refnum"=w873) -> ("refnum out"=w874:T2)  [unwired: 1 in, 6 out]
          }
          frame "double" {
            n365 = Variant To Data(type=0.0 ("Signal"), Variant=w884) -> (data=w885:dbl)  [unwired: 1 in, 1 out]
            n366 = call-poly <vilib>:"Write Key.vi"("section"=w882, "value"=w885, "key"=w883, "refnum"=w880) -> ("refnum out"=w881:T2)  [unwired: 4 in, 3 out]
          }
          frame "int" {
            n367 = Variant To Data(type=u32 0 ("Signal"), Variant=w889) -> (data=w892:u32)  [unwired: 1 in, 1 out]
            n368 = call-poly <vilib>:"Write Key.vi"("section"=w891, "value"=w892, "key"=w890, "refnum"=w887) -> ("refnum out"=w888:T2)  [unwired: 1 in, 6 out]
          }
          frame "string" {
            n369 = Variant To Data(type="", Variant=w898) -> (data=w899:string)  [unwired: 1 in, 1 out]
            n370 = call-poly <vilib>:"Write Key.vi"("section"=w897, "value"=w899, "key"=w896, "refnum"=w894) -> ("refnum out"=w895:T2)  [unwired: 2 in, 5 out]
          }
          frame "enum" {
            n371 = Variant To Data(type=enum16{""}."", Variant=w906) -> (data=w909:enum16{""})  [unwired: 1 in, 1 out]
            n372 = Format Into String(format string="%s", w909) -> (resulting string=w907:string)  [unwired: 2 in, 1 out]
            n373 = call-poly <vilib>:"Write Key.vi"("section"=w904, "value"=w907, "key"=w905, "refnum"=w901) -> ("refnum out"=w902:T2)  [unwired: 2 in, 5 out]
          }
          frame Default {
          }
        }
      }
    }
    frame 5 {
      w920 = i32[] [0, 0, 0, 0, 0, 0, 0, 0]  # Offset
      w919 = i32[] [-1, 1, 1, 1, 1, 1, 1, 1]  # Cal
      w915 = string[] ["m", "V", "V", "V", "V", "V", "V", ""]  # Unit
      w913 = string[] ["Height", "Vert. Deflection", "Horiz. Deflection", "Channel 4", "Channel 5", "Channel 6", "AuxIn", "Obelix"]  # Name
      w921 = "SignalMonitor"  # Section
      # "replace by fgv Signals"
      # "Signal Monitor"
      n374 = for {
        tunnel: w913 -> [w941] mode=indexing
        tunnel: "channel " -> [w940]
        tunnel: w915 -> [w931] mode=indexing
        tunnel: "unit " -> [w938]
        tunnel: "cal " -> [w937]
        tunnel: "offset " -> [w936]
        tunnel: w919 -> [w930] mode=indexing
        tunnel: w920 -> [w929] mode=indexing
        tunnel: w921 -> [w928]
        tunnel: [w924] -> w912
        tunnel: w911 -> [w922]
        i -> [w923]
        n375 = Number To Decimal String(number=w923) -> (decimal integer string=w935:string)  [unwired: 1 in]
        n376 = Concatenate Strings(w940, w935) -> (w939:string)
        n377 = Concatenate Strings(w938, w935) -> (w934:string)
        n378 = Concatenate Strings(w937, w935) -> (w933:string)
        n379 = Concatenate Strings(w936, w935) -> (w932:string)
        n380 = call-poly <vilib>:"Write Key.vi"("section"=w928, "value"=w941, "key"=w939, "refnum"=w922) -> ("refnum out"=w927:T2)  [unwired: 2 in, 5 out]
        n381 = call-poly <vilib>:"Write Key.vi"("section"=w928, "value"=w931, "key"=w934, "refnum"=w927) -> ("refnum out"=w926:T2)  [unwired: 2 in, 5 out]
        n382 = call-poly <vilib>:"Write Key.vi"("section"=w928, "value"=w930, "key"=w933, "refnum"=w926) -> ("refnum out"=w925:T2)  [unwired: 1 in, 6 out]
        n383 = call-poly <vilib>:"Write Key.vi"("section"=w928, "value"=w929, "key"=w932, "refnum"=w925) -> ("refnum out"=w924:T2)  [unwired: 1 in, 6 out]
      }
    }
  }
  n384 = stacked-sequence {
    tunnel: [_ _ _ _ _ _ _ _ w1337] -> w5
    frame #0 {
      w948 = "General"  # Section
      # "General"
      n385 = Get Date/Time In Seconds() -> (seconds since 1Jan1904=w946:timestamp)
      n386 = Format Date/Time String(seconds (now)=w946) -> (date/time string=w947:string)  [unwired: 2 in]
      n387 = call-poly <vilib>:"Write Key.vi"("section"=w948, "value"=w947, "key"="last open") -> ("refnum out"=w945:T2)  [unwired: 3 in, 5 out]
      n388 = call-poly <vilib>:"Write Key.vi"("section"=w948, "value"="Generic 1 (FPGA RIO0, USB-7856 OEM)", "key"="Software version", "refnum"=w945) -> ()  [unwired: 2 in, 6 out]
    }
    frame #1 {
      w952 = "WindowPositions"  # Section
      # "problem fenêtre monitor.vit"
      # "Window Positions"
      n389 = disable-structure shown="Enabled" {
        disable-tunnel: [string[] ["Menu.vi", "Calibration.vi", "Excitation.vi", "Monitor.vit", "Oscilloscope.vi", "Ramp.vi", "Scan.vi", "Signals.vi", "ZController.vi", "4xMonitor.vi", "3xMonitor.vi"] _] -> w949
        frame Enabled {
        }
        frame Disabled {
        }
      }
      n390 = call <vilib>:"Application Directory.vi"() -> ("Application Directory"=w951:path)
      n391 = for {
        tunnel: "FrontPanel\\" ("string") -> [w961]
        tunnel: w951 -> [w958]
        tunnel: w949 -> [w957] mode=indexing
        tunnel: w952 -> [w956]
        # "0 0 Standard/Closed"
        n392 = Concatenate Strings(w961, w957) -> (w960:string)
        n393 = Build Path(base path=w958, name or relative path=w960) -> (appended path=w959:path)
        n394 = Open VI Reference(vi path=w959) -> (vi reference=w955:refnum<vi>, error out=w954:errorcluster)  [unwired: 5 in]
        n395 = case shown="No Error" w954 {
          tunnel: w957 -> [w968 _]
          tunnel: w956 -> [w967 _]
          tunnel: w955 -> [w966 _]
          frame No Error {
            n396 = property class="VI"(reference=w966) -> ("Panel"=w975:refnum<vi>, "FP.State"=w965:T8)  [unwired: 1 in, 2 out]
            n397 = Format Into String(format string="%s", w965) -> (resulting string=w962:string)  [unwired: 2 in, 1 out]
            n398 = property class="Pnl"(reference=w975) -> ("Position"=w974:T9)  [unwired: 1 in, 2 out]
            n399 = Unbundle By Name(w974) -> ("Left"=w973:i32, "Top"=w972:i32)
            n400 = Number To Decimal String(number=w973) -> (decimal integer string=w971:string)  [unwired: 1 in]
            n401 = Number To Decimal String(number=w972) -> (decimal integer string=w970:string)  [unwired: 1 in]
            n402 = call <vilib>:"Space Constant.vi"() -> ("String"=w963:string)
            n403 = Concatenate Strings(w971, w963, w970, w963, w962) -> (w969:string)
            n404 = call-poly <vilib>:"Write Key.vi"("section"=w967, "value"=w969, "key"=w968) -> ()  [unwired: 3 in, 6 out]
          }
          frame Error {
          }
        }
      }
    }
    frame #2 {
      w992 = "PiezoCal"  # Section
      # "PiezoCal"
      n405 = disable-structure shown="Disabled" {
        disable-tunnel: [string[] [": Sensitivity X (m/V)", ": Range X (m)", ": Gain X", ": Sensitivity Y (m/V)", ": Range Y (m)", ": Gain Y", ": Sensitivity Z (m/V)", ": Range Z (m)", ": Gain Z"] ("Array") _] -> _
        frame Disabled {
          (unwired) string[] [": Sensitivity X (m/V)", ": Range X (m)", ": Gain X"] ("Array")
          (unwired) string[] [": Sensitivity Z (m/V)", ": Range Z (m)", ": Gain Z"] ("Array")
          (unwired) string[] [": Sensitivity Y (m/V)", ": Range Y (m)", ": Gain Y"] ("Array")
        }
        frame Enabled {
        }
      }
      n406 = call "FGVCalibrations.vi"("Enum"=Enum."Read") -> ("calibOut"=w984:T10)  [unwired: 9 in, 1 out]
      n407 = Unbundle By Name(w984) -> ("calibIndex"=w994:i32, "calibName"=w980:string[], "calibParameters"=w993:T11)
      n408 = call-poly <vilib>:"Write Key.vi"("section"=w992, "value"=w994, "key"="active calib.") -> ("refnum out"=w991:T2)  [unwired: 5 in, 3 out]
      n409 = call-poly <vilib>:"Write Key.vi"("section"=w992, "key"="hysteresis fast", "refnum"=w991) -> ("refnum out"=w990:T2)  [unwired: 2 in, 6 out]
      n410 = call-poly <vilib>:"Write Key.vi"("section"=w992, "key"="hysteresis slow", "refnum"=w990) -> ("refnum out"=w989:T2)  [unwired: 2 in, 6 out]
      n411 = call-poly <vilib>:"Write Key.vi"("section"=w992, "key"="hysteresis compensation ", "refnum"=w989) -> ("refnum out"=w982:T2)  [unwired: 2 in, 6 out]
      n412 = Array Size(array=w980) -> (size(s)=w981:i32)
      n413 = Build Array(string[] [": Sensitivity X (m/V)", ": Range X (m)", ": Gain X"] ("Array"), string[] [": Sensitivity Y (m/V)", ": Range Y (m)", ": Gain Y"] ("Array"), string[] [": Sensitivity Z (m/V)", ": Range Z (m)", ": Gain Z"] ("Array")) -> (w979:string[][])
      n414 = for {
        N: w981 -> [_]
        tunnel: w993 -> [w1001]
        tunnel: w979 -> [w1000]
        tunnel: w992 -> [w999]
        tunnel: w980 -> [w997]
        tunnel: w982 -> [w998]
        i -> [w996]
        n415 = for {
          tunnel: w997 -> [w1023]
          tunnel: w1001 -> [w1019]
          tunnel: w999 -> [w1017]
          tunnel: w1000 -> [w1002] mode=indexing
          tunnel: w998 -> [w1009]
          tunnel: w996 -> [w1007]
          tunnel: w996 -> [w1006]
          i -> [w1005]
          w1004 = "calib."
          n416 = Index Array(array=w1023, index=w1006) -> (element=w1020:string)
          n417 = Index Array(array=w1019, index=w1005) -> (element=w1018:T12)
          n418 = Number To Decimal String(number=w1007) -> (decimal integer string=w1003:string)  [unwired: 1 in]
          n419 = Unbundle By Name(w1018) -> ("Sensitivity"=w1016:T13, "Range"=w1014:T14, "HV gain"=w1015:T15)
          n420 = Concatenate Strings(w1004, w1003, ": Name") -> (w1021:string)
          n421 = Cluster To Array(cluster=w1016) -> (array=w1013:dbl[])
          n422 = Cluster To Array(cluster=w1014) -> (array=w1012:dbl[])
          n423 = Cluster To Array(cluster=w1015) -> (array=w1011:dbl[])
          n424 = Build Array (concatenate)(w1013, w1012, w1011) -> (w1010:dbl[])
          n425 = call-poly <vilib>:"Write Key.vi"("section"=w1017, "value"=w1020, "key"=w1021, "refnum"=w1009) -> ("refnum out"=w1008:T2)  [unwired: 2 in, 5 out]
          n426 = for {
            tunnel: [w1024] -> _ mode=indexing
            tunnel: w1017 -> [w1030]
            tunnel: w1010 -> [w1029] mode=indexing
            tunnel: w1008 -> [w1028]
            tunnel: w1004 -> [w1027]
            tunnel: w1003 -> [w1026]
            tunnel: w1002 -> [w1025] mode=indexing
            n427 = Concatenate Strings(w1027, w1026, w1025) -> (w1024:string)
            n428 = call-poly <vilib>:"Write Key.vi"("section"=w1030, "value"=w1029, "key"=w1024, "refnum"=w1028) -> ()  [unwired: 4 in, 4 out]
          }
        }
      }
    }
    frame #3 {
      w1051 = "Z-Controller"  # Section
      # "Z-Controller"
      n429 = call "FGVCalibrations.vi"("Enum"=Enum."Read") -> ("calibOut"=w1054:T10)  [unwired: 9 in, 1 out]
      n430 = Unbundle By Name(w1054) -> ("calibParameters"=w1055:T11, "calibIndex"=w1056:i32)
      n431 = Index Array(array=w1055, index=w1056) -> (element=w1035:T12)
      n432 = Unbundle By Name(w1035) -> ("Range.Range Z"=w1034:dbl)
      n433 = Divide(x=w1034, y=2.0) -> (x/y=w1060:dbl)
      n434 = for {
        tunnel: string[] ["Z:min (m)", "Z:max (m)"] -> [w1169] mode=indexing
        tunnel: w1060 -> [w1167]
        tunnel: w1051 -> [w1166]
        tunnel: [w1165] -> w1039
        tunnel: T4."engineering" ("format (fractional)") -> [w1164]
        tunnel: [w1164] -> w1031
        i -> [w1171]
        n435 = Negate(x=w1167) -> (-x=w1168:dbl)
        n436 = Equal?(x=0, y=w1171) -> (x = y?=w1172:bool)
        n437 = Select(t=w1167, s=w1172, f=w1168) -> (s? t:f=w1173:dbl)
        n438 = call-poly <vilib>:"Write Key.vi"("format (fractional)"=w1164, "section"=w1166, "value"=w1173, "key"=w1169) -> ("refnum out"=w1165:T2)  [unwired: 4 in, 3 out]
      }
      n439 = for {
        tunnel: string[] ["Z High Limit", "Z Low limit"] -> [w1159] mode=indexing
        tunnel: w1060 -> [w1157]
        tunnel: w1051 -> [w1156]
        tunnel: [w1155] -> w1048
        tunnel: w1039 -> [w1154]
        tunnel: [w1153] -> w1045
        tunnel: w1031 -> [w1152]
        i -> [w1161]
        n440 = Equal?(x=0, y=w1161) -> (x = y?=w1162:bool)
        n441 = Negate(x=w1157) -> (-x=w1158:dbl)
        n442 = Select(t=w1157, s=w1162, f=w1158) -> (s? t:f=w1163:dbl)
        n443 = call-poly <vilib>:"Write Key.vi"("format (fractional)"=w1152, "section"=w1156, "value"=w1163, "key"=w1159, "refnum"=w1154) -> ("error out"=w1153:errorcluster, "refnum out"=w1155:T2)  [unwired: 3 in, 2 out]
      }
      n444 = call "FGVController.vi"("Enum"=Enum."Read") -> ("ManualMotionDecOut"=w1043:cluster{"WithdrawDec":u16, "ManualMoveDec":u16}, "calibOut"=w1041:T16, "liftHeightOut"=w1050:dbl)  [unwired: 6 in, 2 out]
      n445 = Unbundle By Name(w1041) -> ("ActiveController"=w1057:dbl, "ControllerParameters"=w1058:T17)  [unwired: 1 out]
      n446 = Cluster To Array(cluster=w1043) -> (array=w1044:u16[])
      n447 = call-poly <vilib>:"Write Key.vi"("format (fractional)"=w1031, "section"=w1051, "error in (no error)"=w1045, "value"=w1050, "key"="liftHeight", "refnum"=w1048) -> ("error out"=w1046:errorcluster, "refnum out"=w1047:T2)  [unwired: 2 in, 2 out]
      n448 = for {
        tunnel: w1051 -> [w1093]
        tunnel: w1047 -> [w1092]
        tunnel: w1046 -> [w1091]
        tunnel: string[] ["manual move decimation", "withdraw decimation"] -> [w1090] mode=indexing
        tunnel: w1044 -> [w1089] mode=indexing
        tunnel: [w1088] -> _
        tunnel: [w1087] -> w1033
        n449 = call-poly <vilib>:"Write Key.vi"("section"=w1093, "error in (no error)"=w1091, "value"=w1089, "key"=w1090, "refnum"=w1092) -> ("error out"=w1088:errorcluster, "refnum out"=w1087:T2)  [unwired: 3 in, 2 out]
      }
      n450 = for {
        tunnel: w1058 -> [w1086] mode=indexing
        tunnel: w1057 -> [w1064]
        tunnel: [w1061] -> w1052 mode=indexing
        i -> [w1065]
        n451 = Unbundle(w1086) -> ("Controller Config"=w1085:T18, "PID"=w1084:T19)
        n452 = Unbundle By Name(w1085) -> ("Controller name"=w1083:string, "Control Signal name"=w1082:string, "Unit"=w1081:string, "Controller type"=w1080:enum16{"Bipolar", "Absolute"}, "Signal"=w1079:T5, "Slope"=w1078:bool)
        n453 = Unbundle By Name(w1084) -> ("Setpoint"=w1077:dbl, "I Gain"=w1076:dbl, "P Gain"=w1075:dbl)
        n454 = Equal?(x=w1064, y=w1065) -> (x = y?=w1063:bool)
        n455 = To Variant(anything=w1083) -> (Variant=w1074:variant)
        n456 = To Variant(anything=w1082) -> (Variant=w1073:variant)
        n457 = To Variant(anything=w1081) -> (Variant=w1072:variant)
        n458 = To Variant(anything=w1080) -> (Variant=w1071:variant)
        n459 = To Variant(anything=w1079) -> (Variant=w1070:variant)
        n460 = To Variant(anything=w1078) -> (Variant=w1069:variant)
        n461 = To Variant(anything=w1077) -> (Variant=w1068:variant)
        n462 = To Variant(anything=w1076) -> (Variant=w1067:variant)
        n463 = To Variant(anything=w1075) -> (Variant=w1066:variant)
        n464 = To Variant(anything=w1063) -> (Variant=w1062:variant)
        n465 = Build Array(w1074, w1062, w1073, w1072, w1071, w1070, w1069, w1068, w1067, w1066) -> (w1061:variant[])
      }
      n466 = for {
        tunnel: string[][] [[": Name", "string"], [": Controller on/off", "boolean"], [": Control Signal Name", "string"], [": Unit", "string"], [": Type", "enum"], [": Signal", "int"], [": Slope pos/neg", "boolean"], [": GainScale", "double"], [": Setpoint", "double"], [": Integral :value", "double"], [": Proportional:value", "double"]] ("appended array") -> [w1102]
        tunnel: w1052 -> [w1097] mode=indexing
        tunnel: w1051 -> [w1099]
        tunnel: w1033 -> [w1095]
        tunnel: [w1096] -> _
        i -> [w1094]
        n467 = Index Array(array=w1102, index (row) #1=w1094, index (col) #1=0 ("disabled index (col)"), index (row) #2=w1094, index (col) #2=1 ("disabled index (col)")) -> (element #1=w1104:string, element #2=w1100:string)
        n468 = Number To Decimal String(number=w1094) -> (decimal integer string=w1105:string)  [unwired: 1 in]
        n469 = Concatenate Strings("controller.", w1105, w1104) -> (w1098:string)
        n470 = for {
          tunnel: w1100 -> [w1112]
          tunnel: w1099 -> [w1111]
          tunnel: w1098 -> [w1110]
          tunnel: w1097 -> [w1109] mode=indexing
          tunnel: w1095 -> [w1107]
          tunnel: [w1108] -> w1096
          n471 = case shown="\"double\"" w1112 {
            tunnel: w1111 -> [w1116 w1123 w1130 w1141 w1150 _]
            tunnel: w1110 -> [w1115 w1124 w1131 w1140 w1149 _]
            tunnel: w1109 -> [w1119 w1126 w1133 w1137 w1148 _]
            tunnel: [w1113 w1121 w1129 w1136 w1142 w1151] -> w1108
            tunnel: w1107 -> [w1114 w1122 w1128 w1135 w1143 w1151]
            frame "boolean" {
              n472 = Variant To Data(type=TRUE, Variant=w1119) -> (data=w1117:bool)  [unwired: 1 in, 1 out]
              n473 = call-poly <vilib>:"Write Key.vi"("section"=w1116, "value"=w1117, "key"=w1115, "refnum"=w1114) -> ("refnum out"=w1113:T2)  [unwired: 1 in, 6 out]
            }
            frame "double" {
              n474 = Variant To Data(type=0.0 ("Signal"), Variant=w1126) -> (data=w1125:dbl)  [unwired: 1 in, 1 out]
              n475 = call-poly <vilib>:"Write Key.vi"("format (fractional)"=T4."engineering", "section"=w1123, "value"=w1125, "key"=w1124, "refnum"=w1122) -> ("refnum out"=w1121:T2)  [unwired: 3 in, 3 out]
            }
            frame "int" {
              n476 = Variant To Data(type=u16 0 ("Signal"), Variant=w1133) -> (data=w1132:u16)  [unwired: 1 in, 1 out]
              n477 = call-poly <vilib>:"Write Key.vi"("section"=w1130, "value"=w1132, "key"=w1131, "refnum"=w1128) -> ("refnum out"=w1129:T2)  [unwired: 1 in, 6 out]
            }
            frame "string" {
              n478 = Variant To Data(type="", Variant=w1137) -> (data=w1138:string)  [unwired: 1 in, 1 out]
              n479 = call-poly <vilib>:"Write Key.vi"("section"=w1141, "value"=w1138, "key"=w1140, "refnum"=w1135) -> ("refnum out"=w1136:T2)  [unwired: 2 in, 5 out]
            }
            frame "enum" {
              n480 = Variant To Data(type=T5."..." ("Signal"), Variant=w1148) -> (data=w1146:T5)  [unwired: 1 in, 1 out]
              n481 = Format Into String(format string="%s", w1146) -> (resulting string=w1144:string)  [unwired: 2 in, 1 out]
              n482 = call-poly <vilib>:"Write Key.vi"("section"=w1150, "value"=w1144, "key"=w1149, "refnum"=w1143) -> ("refnum out"=w1142:T2)  [unwired: 2 in, 5 out]
            }
            frame Default {
            }
          }
        }
      }
    }
    frame #4 {
      w1176 = "Motor Control Step"  # Section
      # "Motor Control Step"
      n483 = for {
        tunnel: string[] ["motor speed (rpm)", "steps per click", "step size", "step up direction", "line A", "line B", "line C", "line D"] -> [w1180] mode=indexing
        tunnel: i32[] [1000, 5, 5, 1, 1, 2, 3, 4] ("number") -> [w1179] mode=indexing
        tunnel: w1176 -> [w1178]
        tunnel: [w1177] -> _
        n484 = call-poly <vilib>:"Write Key.vi"("section"=w1178, "value"=w1179, "key"=w1180) -> ("refnum out"=w1177:T2)  [unwired: 2 in, 6 out]
      }
    }
    frame #5 {
      w1184 = "XY-Waveforms"  # Section
      # "XY-Waveforms"
      n485 = call "FGVScanWaveform.vi"("Enum"=Enum."Read") -> ("scanWaveFormCtl Out"=w1201:T21)  [unwired: 9 in, 1 out]
      n486 = Unbundle By Name(w1201) -> ("fastWavePts"=w1200:u16, "fastRoundPts"=w1199:u16, "fastWaveType"=w1197:T20, "slowWavePts"=w1183:u16, "slowRoundPts"=w1182:u16, "slowWaveType"=w1181:T20)
      n487 = Build Array(w1200, w1199) -> (w1198:u16[])
      n488 = for {
        tunnel: w1198 -> [w1211] mode=indexing
        tunnel: string[] ["Fast Wave Pts", "Fast Round Pts"] -> [w1210] mode=indexing
        tunnel: w1184 -> [w1209]
        tunnel: [w1208] -> w1195
        n489 = call-poly <vilib>:"Write Key.vi"("section"=w1209, "value"=w1211, "key"=w1210) -> ("refnum out"=w1208:T2)  [unwired: 2 in, 6 out]
      }
      n490 = Build Array(w1183, w1182) -> (w1186:u16[])
      n491 = Format Into String(format string="%s", w1197) -> (resulting string=w1194:string)  [unwired: 2 in, 1 out]
      n492 = call-poly <vilib>:"Write Key.vi"("section"=w1184, "value"=w1194, "key"="Fast Wave Type", "refnum"=w1195) -> ("refnum out"=w1187:T2)  [unwired: 2 in, 5 out]
      n493 = for {
        tunnel: w1186 -> [w1207] mode=indexing
        tunnel: string[] ["Slow Wave Pts", "Slow Round Pts"] -> [w1206] mode=indexing
        tunnel: w1184 -> [w1205]
        tunnel: [w1204] -> w1189
        tunnel: w1187 -> [w1203]
        n494 = call-poly <vilib>:"Write Key.vi"("section"=w1205, "value"=w1207, "key"=w1206, "refnum"=w1203) -> ("refnum out"=w1204:T2)  [unwired: 1 in, 6 out]
      }
      n495 = Format Into String(format string="%s", w1181) -> (resulting string=w1190:string)  [unwired: 2 in, 1 out]
      n496 = call-poly <vilib>:"Write Key.vi"("section"=w1184, "value"=w1190, "key"="Slow Wave Type", "refnum"=w1189) -> ()  [unwired: 2 in, 6 out]
    }
    frame #6 {
      w1215 = string[][] [["width", "double"], ["height", "double"], ["x offset", "double"], ["y offset", "double"], ["angle", "double"], ["pixels/line", "int"], ["lines", "int"], ["time/line", "double"], ["scan rate", "double"], ["single scan direction", "boolean"], ["autosave", "boolean"], ["Filename", "string"], ["Folder", "path"]] ("transposed array")
      w1238 = "Scan"  # Section
      # "read autosave\nFilename\nFolder"
      # "autosave"
      # "Scan"
      n497 = call "FGVScanParameters.vi"("Enum"=Enum."Read") -> ("Scan Parameters Out"=w1218:T22)  [unwired: 9 in, 1 out]
      n498 = call "FGVScanWaveform.vi"("Enum"=Enum."Read") -> ("scanWaveFormCtl Out"=w1240:T21)  [unwired: 9 in, 1 out]
      n499 = call "FGVSavingParameters.vi"("Enum"=Enum."Read") -> ()  [unwired: 7 in, 4 out]
      n500 = Unbundle By Name(w1218) -> ("Width"=w1228:dbl, "Height"=w1229:dbl, "X Offset"=w1230:dbl, "Y Offset"=w1231:dbl, "Angle"=w1232:dbl, "Pixels/Line"=w1233:u16, "Lines"=w1234:u16, "Time/Line"=w1235:dbl, "Scan Rate"=w1236:dbl)
      n501 = Unbundle By Name(w1240) -> ("singleDirectionScan"=w1241:bool)
      n502 = To Variant(anything=w1228) -> (Variant=w1219:variant)
      n503 = To Variant(anything=w1229) -> (Variant=w1227:variant)
      n504 = To Variant(anything=w1230) -> (Variant=w1220:variant)
      n505 = To Variant(anything=w1231) -> (Variant=w1221:variant)
      n506 = To Variant(anything=w1232) -> (Variant=w1222:variant)
      n507 = To Variant(anything=w1233) -> (Variant=w1223:variant)
      n508 = To Variant(anything=w1234) -> (Variant=w1224:variant)
      n509 = To Variant(anything=w1235) -> (Variant=w1225:variant)
      n510 = To Variant(anything=w1236) -> (Variant=w1226:variant)
      n511 = To Variant(anything=path "C:/") -> (Variant=w1248:variant)
      n512 = To Variant(anything=TRUE) -> (Variant=w1246:variant)
      n513 = To Variant(anything="Filename") -> (Variant=w1247:variant)
      n514 = To Variant(anything=w1241) -> (Variant=w1242:variant)
      n515 = Build Array(w1219, w1227, w1220, w1221, w1222, w1223, w1224, w1225, w1226, w1242, w1246, w1247, w1248) -> (w1237:variant[])
      n516 = Array Size(array=w1215) -> (size(s)=w1214:i32[])
      n517 = Index Array(array=w1214, index=0) -> (element=w1213:i32)
      n518 = for {
        N: w1213 -> [_]
        tunnel: w1215 -> [w1254]
        tunnel: w1237 -> [w1256] mode=indexing
        tunnel: w1238 -> [w1255]
        i -> [w1251]
        n519 = Index Array(array=w1254, index (row) #1=w1251, index (col) #1=0 ("disabled index (col)"), index (row) #2=w1251, index (col) #2=1 ("disabled index (col)")) -> (element #1=w1252:string, element #2=w1249:string)
        n520 = case shown="\"double\"" w1249 {
          tunnel: w1256 -> [w1259 w1265 w1270 w1275 w1280 _]
          tunnel: w1255 -> [w1258 w1264 w1269 w1273 w1279 _]
          tunnel: w1252 -> [w1257 w1263 w1268 w1274 w1278 _]
          frame "boolean" {
            n521 = Variant To Data(type=TRUE, Variant=w1259) -> (data=w1260:bool)  [unwired: 1 in, 1 out]
            n522 = call-poly <vilib>:"Write Key.vi"("section"=w1258, "value"=w1260, "key"=w1257) -> ()  [unwired: 2 in, 7 out]
          }
          frame "double" {
            n523 = Variant To Data(type=0.0 ("Signal"), Variant=w1265) -> (data=w1266:dbl)  [unwired: 1 in, 1 out]
            n524 = call-poly <vilib>:"Write Key.vi"("format (fractional)"=T4."engineering", "section"=w1264, "value"=w1266, "key"=w1263) -> ()  [unwired: 4 in, 4 out]
          }
          frame "int" {
            n525 = Variant To Data(type=u32 0 ("Signal"), Variant=w1270) -> (data=w1271:u32)  [unwired: 1 in, 1 out]
            n526 = call-poly <vilib>:"Write Key.vi"("section"=w1269, "value"=w1271, "key"=w1268) -> ()  [unwired: 2 in, 7 out]
          }
          frame "string" {
            n527 = Variant To Data(type="", Variant=w1275) -> (data=w1276:string)  [unwired: 1 in, 1 out]
            n528 = call-poly <vilib>:"Write Key.vi"("section"=w1273, "value"=w1276, "key"=w1274) -> ()  [unwired: 3 in, 6 out]
          }
          frame "enum" {
            n529 = Variant To Data(type=T5."..." ("Signal"), Variant=w1280) -> (data=w1283:T5)  [unwired: 1 in, 1 out]
            n530 = Format Into String(format string="%s", w1283) -> (resulting string=w1281:string)  [unwired: 2 in, 1 out]
            n531 = call-poly <vilib>:"Write Key.vi"("section"=w1279, "value"=w1281, "key"=w1278) -> ()  [unwired: 3 in, 6 out]
          }
          frame Default {
          }
        }
      }
    }
    frame #7 {
      w1288 = string[][] [["Channel", "int"], ["Direction", "enum"], ["Processing", "enum"], ["Color", "enum"], ["noSelection/fullScale/standardDev", "enum"]] ("transposed array")
      w1289 = "ScanMonitor"  # Section
      # "bug enum"
      # "Direction: int--> enum"
      # "Scan Monitor"
      n532 = Unbundle(T7 {0, "Direction"=enum."Forward", "Processing"=enum."None", "Color"=enum."Blue"} ("Controls")) -> (w1295:i32, "Direction"=w1296:enum16{"Forward", "Backward"}, "Processing"=w1297:enum16{"None", "Offset", "Line", "Polynom"}, "Color"=w1298:T23)
      n533 = To Variant(anything=T6."FullScale" ("ZScale")) -> (Variant=w1300:variant)
      n534 = To Variant(anything=w1295) -> (Variant=w1290:variant)
      n535 = To Variant(anything=w1296) -> (Variant=w1293:variant)
      n536 = To Variant(anything=w1297) -> (Variant=w1292:variant)
      n537 = To Variant(anything=w1298) -> (Variant=w1291:variant)
      n538 = Array Size(array=w1288) -> (size(s)=w1286:i32[])
      n539 = Build Array(w1290, w1293, w1292, w1291, w1300) -> (w1299:variant[])
      n540 = Index Array(array=w1286, index=0) -> (element=w1287:i32)
      n541 = for {
        N: w1287 -> [_]
        tunnel: w1288 -> [w1308]
        tunnel: w1289 -> [w1309]
        tunnel: w1299 -> [w1302] mode=indexing
        i -> [w1305]
        (unwired) enum16{"Forward", "Backward"}."Forward" ("Direction")
        n542 = Index Array(array=w1308, index (row) #1=w1305, index (col) #1=0 ("disabled index (col)"), index (row) #2=w1305, index (col) #2=1 ("disabled index (col)")) -> (element #1=w1306:string, element #2=w1303:string)
        n543 = case shown="\"enum\"" w1303 {
          tunnel: w1309 -> [w1311 w1315 w1322 w1326 w1331 _]
          tunnel: w1306 -> [w1310 w1316 w1321 w1325 w1332 _]
          tunnel: w1302 -> [w1312 w1317 w1320 w1327 w1333 _]
          frame "boolean" {
            n544 = Variant To Data(type=TRUE, Variant=w1312) -> (data=w1313:bool)  [unwired: 1 in, 1 out]
            n545 = call-poly <vilib>:"Write Key.vi"("section"=w1311, "value"=w1313, "key"=w1310) -> ()  [unwired: 2 in, 7 out]
          }
          frame "double" {
            n546 = Variant To Data(type=0.0 ("Signal"), Variant=w1317) -> (data=w1318:dbl)  [unwired: 1 in, 1 out]
            n547 = call-poly <vilib>:"Write Key.vi"("section"=w1315, "value"=w1318, "key"=w1316) -> ()  [unwired: 5 in, 4 out]
          }
          frame "int" {
            n548 = Variant To Data(type=u32 0 ("Signal"), Variant=w1320) -> (data=w1323:u32)  [unwired: 1 in, 1 out]
            n549 = call-poly <vilib>:"Write Key.vi"("section"=w1322, "value"=w1323, "key"=w1321) -> ()  [unwired: 2 in, 7 out]
          }
          frame "string" {
            n550 = Variant To Data(type="", Variant=w1327) -> (data=w1328:string)  [unwired: 1 in, 1 out]
            n551 = call-poly <vilib>:"Write Key.vi"("section"=w1326, "value"=w1328, "key"=w1325) -> ()  [unwired: 3 in, 6 out]
          }
          frame "enum" {
            n552 = Variant To Data(type=enum16{""}."", Variant=w1333) -> (data=w1336:enum16{""})  [unwired: 1 in, 1 out]
            n553 = Format Into String(format string="%s", w1336) -> (resulting string=w1334:string)  [unwired: 2 in, 1 out]
            n554 = call-poly <vilib>:"Write Key.vi"("section"=w1331, "value"=w1334, "key"=w1332) -> ()  [unwired: 3 in, 6 out]
          }
          frame Default {
          }
        }
      }
    }
    frame #8 {
      w1345 = i32[] [0, 0, 0, 0, 0, 0, 0, 0]  # Offset
      w1344 = i32[] [-1, 1, 1, 1, 1, 1, 1, 1]  # Cal
      w1340 = string[] ["m", "V", "V", "V", "V", "V", "V", ""]  # Unit
      w1338 = string[] ["Height", "Vert. Deflection", "Horiz. Deflection", "Channel 4", "Channel 5", "Channel 6", "AuxIn", "Obelix"]  # Name
      w1346 = "SignalMonitor"  # Section
      # "replace by fgv Signals"
      # "Signal Monitor"
      n555 = for {
        tunnel: w1338 -> [w1365] mode=indexing
        tunnel: "channel " -> [w1364]
        tunnel: w1340 -> [w1355] mode=indexing
        tunnel: "unit " -> [w1362]
        tunnel: "cal " -> [w1361]
        tunnel: "offset " -> [w1360]
        tunnel: w1344 -> [w1354] mode=indexing
        tunnel: w1345 -> [w1353] mode=indexing
        tunnel: w1346 -> [w1352]
        tunnel: [w1348] -> w1337
        i -> [w1347]
        n556 = Number To Decimal String(number=w1347) -> (decimal integer string=w1359:string)  [unwired: 1 in]
        n557 = Concatenate Strings(w1364, w1359) -> (w1363:string)
        n558 = Concatenate Strings(w1362, w1359) -> (w1358:string)
        n559 = Concatenate Strings(w1361, w1359) -> (w1357:string)
        n560 = Concatenate Strings(w1360, w1359) -> (w1356:string)
        n561 = call-poly <vilib>:"Write Key.vi"("section"=w1352, "value"=w1365, "key"=w1363) -> ("refnum out"=w1351:T2)  [unwired: 3 in, 5 out]
        n562 = call-poly <vilib>:"Write Key.vi"("section"=w1352, "value"=w1355, "key"=w1358, "refnum"=w1351) -> ("refnum out"=w1350:T2)  [unwired: 2 in, 5 out]
        n563 = call-poly <vilib>:"Write Key.vi"("section"=w1352, "value"=w1354, "key"=w1357, "refnum"=w1350) -> ("refnum out"=w1349:T2)  [unwired: 1 in, 6 out]
        n564 = call-poly <vilib>:"Write Key.vi"("section"=w1352, "value"=w1353, "key"=w1356, "refnum"=w1349) -> ("refnum out"=w1348:T2)  [unwired: 1 in, 6 out]
      }
    }
  }
  n565 = call <vilib>:"Close Config Data.vi"("refnum"=w5) -> ("error out"=w6:errorcluster)  [unwired: 2 in, 8 out]
  n566 = call <vilib>:"Simple Error Handler.vi"("error in (no error)"=w6) -> ()  [unwired: 1 in, 8 out]
